vi "NEW数据采集传输系统.vi"() -> ()   [LabVIEW 2016, in "数据传输系统.lvlib"]
uses:
  <vilib>/Utility/miscctls.llb/LVPointTypeDef.ctl
  <vilib>/Utility/error.llb/whitespace.ctl
  <vilib>/Utility/config.llb/Read Key (String).vi
  <vilib>/Utility/config.llb/NI_LVConfig.lvlib
  <vilib>/Averna/Notify Icon/NotifyIcon.llb/NotifyIcon.lvclass
  <vilib>/ptbypt/NI_PtbyPt.lvlib
  <vilib>/Averna/Notify Icon/NotifyIcon.llb/BalloonIcon.ctl
  update/update.lvlib
panel:
  out "数据库打开失败次数":dbl
  out "与工控通信指示灯":bool
  in  "判断数据反馈":enum16{"非严格判断", "严格判断", "不判断"}(ring)
  in  "暂停上传":bool
  in  "参数数值":T1={"CODMn"=TRUE, "CODCr"=TRUE, "DO"=TRUE, "铜"=TRUE, "PH"=TRUE, "氨氮"=TRUE, "比电导率"=TRUE, "水温"=TRUE, "COD"=TRUE, "浊度"=TRUE, "总氮"=TRUE, "总磷"=TRUE, "叶绿素a"=TRUE, "藻密度"=TRUE, "水位"=TRUE, "流速"=TRUE, "瞬时流量"=TRUE, "累积流量"=TRUE, "亚硝氮"=TRUE, "硫化物"=TRUE, "ORP"=TRUE, "铅"=TRUE, "镉"=TRUE, "锌"=TRUE, "镍"=TRUE, "锰"=TRUE, "汞"=TRUE, "气温"=TRUE, "气压"=TRUE, "风速"=TRUE, "风向"=TRUE}
  in  "配置表":bool caption="确定"
  out "配置表格":string[][](table)
  in  "updateconfiguration":T2={"主机"="27.154.58.30", "用户"="update", "密码"="std23506", "远程路径"="数据传输系统\\平台数据传输系统.exe", "下载文件名"="平台数据传输系统.exe", "软件版本"=""}
  out "标题显示":string
  in  "更新":bool
  out "错误输出":errorcluster
  in  "系统编码选择框":string(combo)="地表水质量监测"
  in  "数据发送通道":enum16{"TCP", "VISA"}(ring)
  in  "baud rate":u32=9600 caption="波特率"
  in  "VISA resource name":refnum<visa-resource-name> caption="VISA资源名称"
  in  "实时数据发送时间间隔/min":i32=1
  in  "数据组合发送":bool
  in  "2011发送":bool
  in  "数据发送协议":enum16{"2005-212协议", "2017-212协议"}(ring)=enum."2017-212协议"
  in  "重发时间":T3(ring)
  in  "重发日期":T4(ring)
  in  "开机启动":bool
  in  "确定更改起始时间":bool
  in  "更改起始时间":bool
  in  "数据发送起始时间":timestamp format="%<%.3X\n%Y/%m/%d>T"
  in  "每周自动重发":bool=TRUE
  in  "确定":bool
  in  "返回":bool
  in  "PW":string
  in  "MN":string
  in  "PORT":string
  in  "IP":string
  in  "站点设备":string
  in  "站点名称":string
  out "设置超时时间/min":i32=1
  out "状态信息":T5={"1st Error to Convert "=63, "步骤 "=enum."发送数据", "元素"="实时数据", "TCP服务端掉线计数"=0, "TCP掉线时间节点"="2019/05/08 15:24:17"} {"1st Error to Convert" items=["无错误", "参数错误", "内存已满", "超出区域", "文件结束", "文件已打开", "一般文件IO错误", "未找到文件", "文件权限错误", "磁盘已满", "路径副本", "打开过多文件", "未启用", "未找到资源文件", "无法添加资源", "未找到资源", "未找到图像", "图像内存错误", "画笔不存在", "配置错误类型", "配置未找到解析段", "配置解析错误", "配置内存错误", "错误外部代码格式", "错误外部代码偏移量", "外部代码不存在", "空窗口", "销毁窗口错误", "空菜单", "打印已中止", "错误打印记录", "打印驱动程序错误", "打印时窗口错误", "打印时内存错误", "打印对话框错误", "一般打印错误", "无效设备引用句柄", "设备未找到", "设备参数错误", "设备单位错误", "无法打开设备", "设备调用已中止", "一般错误", "用户已取消", "对象ID过低", "对象ID过高", "对象不在堆中", "未知的堆", "错误DefProc ID", "DefProc不在表格中", "范围外信息", "空方法", "未知信息", "不支持管理器调用", "错误地址", "连接过程中", "连接超时", "连接过程中", "不支持网络属性", "网络错误", "正在使用的地址", "系统缺少内存", "连接已中止", "连接已拒绝", "连接未建立", "连接已建立", "连接已关闭", "初始化错误（交互应用程序管理器）", "错误事件发生", "等待无约束事件发生处理程序", "事件发生队列溢出", "错误路径", "未发出信号量", "未识别类型（交互应用程序管理器）"]}
  out "数据接收超时指示灯":bool
  out "空闲时间/s":string
  out "系统时间":string
  out "实时小时数据上传":bool
  out "系统状态改变":bool
  out "软件版本":string
  out "掉线指示":bool
  out "核查数据上传":bool
  out "配置信息":T6
  in  "参数配置":bool
  out "反控数据发送":bool
  out "读取报文显示":string
  out "发送报文显示":string
  out "心跳包":bool
  out "通信状态":bool
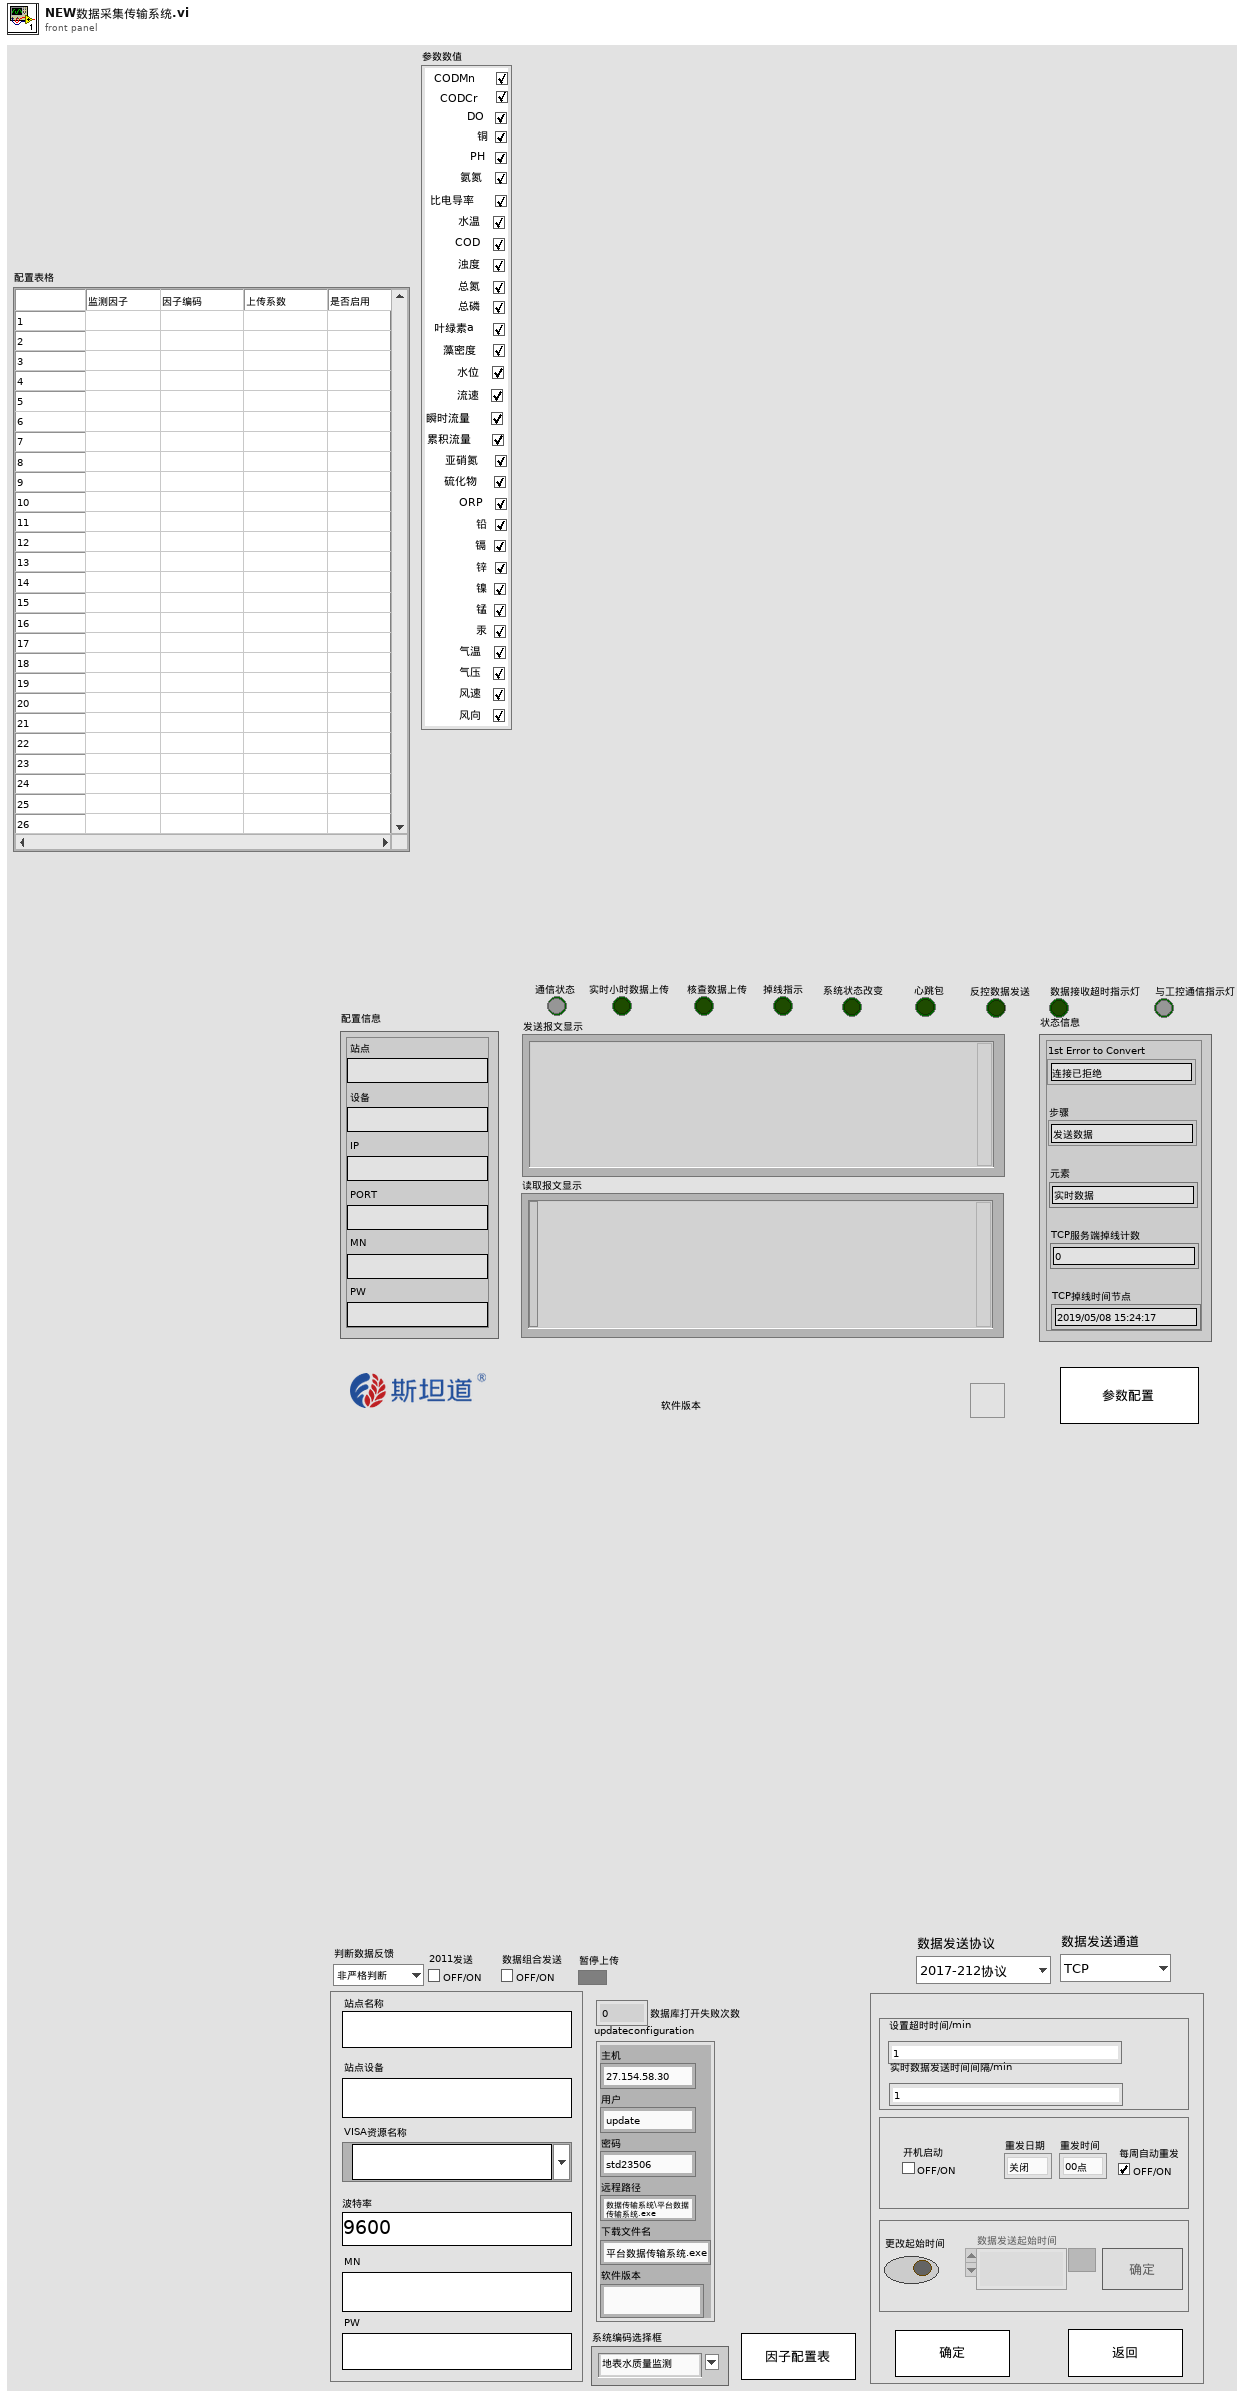
[diagram p1: front panel]
types:
  T1 = cluster{"CODMn":bool, "CODCr":bool, "DO":bool, "铜":bool, "PH":bool, "氨氮":bool, "比电导率":bool, "水温":bool, "COD":bool, "浊度":bool, "总氮":bool, "总磷":bool, "叶绿素a":bool, "藻密度":bool, "水位":bool, "流速":bool, "瞬时流量":bool, "累积流量":bool, "亚硝氮":bool, "硫化物":bool, "ORP":bool, "铅":bool, "镉":bool, "锌":bool, "镍":bool, "锰":bool, "汞":bool, "气温":bool, "气压":bool, "风速":bool, "风向":bool}
  T2 = cluster{"主机":string, "用户":string, "密码":string, "远程路径":string, "下载文件名":string, "软件版本":string}
  T3 = enum16{"00点", "01点", "02点", "03点", "04点", "05点", "06点", "07点", "08点", "09点", "10点", "11点", "12点", "13点", "14点", "15点", "16点", "17点", "18点", "19点", "20点", "21点", "22点", "23点"}
  T4 = enum16{"关闭", "星期日", "星期一", "星期二", "星期三", "星期四", "星期五", "星期六"}
  T5 = cluster{"1st Error to Convert ":i32, "步骤 ":enum16{"打开连接", "发送数据", "读取数据", "数据处理", "关闭连接"}, "元素":string, "TCP服务端掉线计数":i32, "TCP掉线时间节点":string}
  T6 = cluster{"站点":string, "设备":string, "IP":string, "PORT":string, "MN":string, "PW":string}
  T7 = cluster{"host":string, "port":u16, "user":string, "password":string, "远端地址":string}
  T8 = typedef "LVDateTimeRec.ctl" = cluster{"秒数的小数部分":dbl, "秒":i32, "分":i32, "时":i32, "日":i32, "月":i32, "年":i32, "天数（周）":i32, "天数（年）":i32, "DST":i32}
  T9 = typedef "whitespace.ctl" = u16
  T10 = typedef "LVPointTypeDef.ctl" = cluster{"Horizontal":i16, "Vertical":i16}
  T11 = cluster{"setini":string, "sysini":string, "hechaini":string, "actualwrite":string, "actualread":string, "datasent":string, "反控命令信息队列":string, "反控与仪器交互":string}
  T12 = cluster{"CODMn":string, "CODCr":string, "DO":string, "铜":string, "PH":string, "氨氮":string, "比电导率":string, "水温":string, "COD":string, "浊度":string, "总氮":string, "总磷":string, "叶绿素a":string, "藻密度":string, "水位":string, "流速":string, "瞬时流量":string, "累积流量":string, "亚硝酸盐":string, "硫化物":string, "ORP":string, "铅":string, "镉":string, "锌":string, "镍":string, "锰":string, "汞":string, "气温":string, "气压":string, "风速":string, "风向":string}
  T13 = typedef "NI_LVConfig.lvlib/Config Data RefNum.ctl" = refnum<k1>
  T14 = typedef "imagedata.ctl" = cluster{"image type":i32, "image depth":i32, "image":u8[], "mask":u8[], "colors":u32[], "Rectangle":cluster{"left":i16, "top":i16, "right":i16, "bottom":i16}}
  T15 = cluster{"[0]":string, "[1]":string, "[2]":string, "[3]":string, "[4]":string, "[5]":string, "[6]":string, "[7]":string, "[8]":string, "[9]":string, "[10]":string, "[11]":string, "[12]":string, "[13]":string, "[14]":string, "[15]":string, "[16]":string, "[17]":string, "[18]":string, "[19]":string, "[20]":string, "[21]":string, "[22]":string, "[23]":string, "[24]":string, "[25]":string, "[26]":string, "[27]":string, "[28]":string, "[29]":string, "[30]":string}
  T16 = enum8{"Enabled", "Disabled", "Disabled and Grayed Out"}
  T17 = cluster{"配置表格[0]":string, "配置表格[1]":string, "配置表格[2]":string, "配置表格[3]":string, "配置表格[4]":string, "配置表格[5]":string, "配置表格[6]":string, "配置表格[7]":string, "配置表格[8]":string, "配置表格[9]":string, "配置表格[10]":string, "配置表格[11]":string, "配置表格[12]":string, "配置表格[13]":string, "配置表格[14]":string, "配置表格[15]":string, "配置表格[16]":string, "配置表格[17]":string, "配置表格[18]":string, "配置表格[19]":string, "配置表格[20]":string, "配置表格[21]":string, "配置表格[22]":string, "配置表格[23]":string, "配置表格[24]":string, "配置表格[25]":string, "配置表格[26]":string, "配置表格[27]":string, "配置表格[28]":string, "配置表格[29]":string, "配置表格[30]":string}
  T18 = cluster{"[0]":dbl, "[1]":dbl, "[2]":dbl, "[3]":dbl, "[4]":dbl, "[5]":dbl, "[6]":dbl, "[7]":dbl, "[8]":dbl, "[9]":dbl, "[10]":dbl, "[11]":dbl, "[12]":dbl, "[13]":dbl, "[14]":dbl, "[15]":dbl, "[16]":dbl, "[17]":dbl, "[18]":dbl, "[19]":dbl, "[20]":dbl, "[21]":dbl, "[22]":dbl, "[23]":dbl, "[24]":dbl, "[25]":dbl, "[26]":dbl, "[27]":dbl, "[28]":dbl, "[29]":dbl, "[30]":dbl}
  T19 = cluster{"[0]":string, "[1]":string, "[2]":string, "[3]":string, "[4]":string, "[5]":string, "[6]":string, "[7]":string, "[8]":string, "[9]":string, "[10]":string, "[11]":string, "[12]":string}
  T20 = cluster{"[0]":string, "[1]":string, "[2]":string, "[3]":string, "[4]":string, "[5]":string, "[6]":string, "[7]":string}
  T21 = cluster{"[0]":string, "[1]":string, "[2]":string, "[3]":string, "[4]":string, "[5]":string, "[6]":string, "[7]":string, "[8]":string, "[9]":string, "[10]":string, "[11]":string, "[12]":string, "[13]":string, "[14]":string}
  T22 = cluster{"[0]":string, "[1]":string, "[2]":string, "[3]":string, "[4]":string}
  T23 = enum32{"Invalid", "Standard", "Closed", "Hidden", "Minimized", "Maximized"}
  T24 = typedef "NotifyIcon.lvlib/NotifyIcon.lvclass/BalloonIcon.ctl" = enum32{"None", "Information", "Warning", "Error"}
  T25 = enum32{"invalid app kind", "Development System", "Run Time System", "Student Edition", "Embedded LabVIEW", "Evaluation", "Custom"}
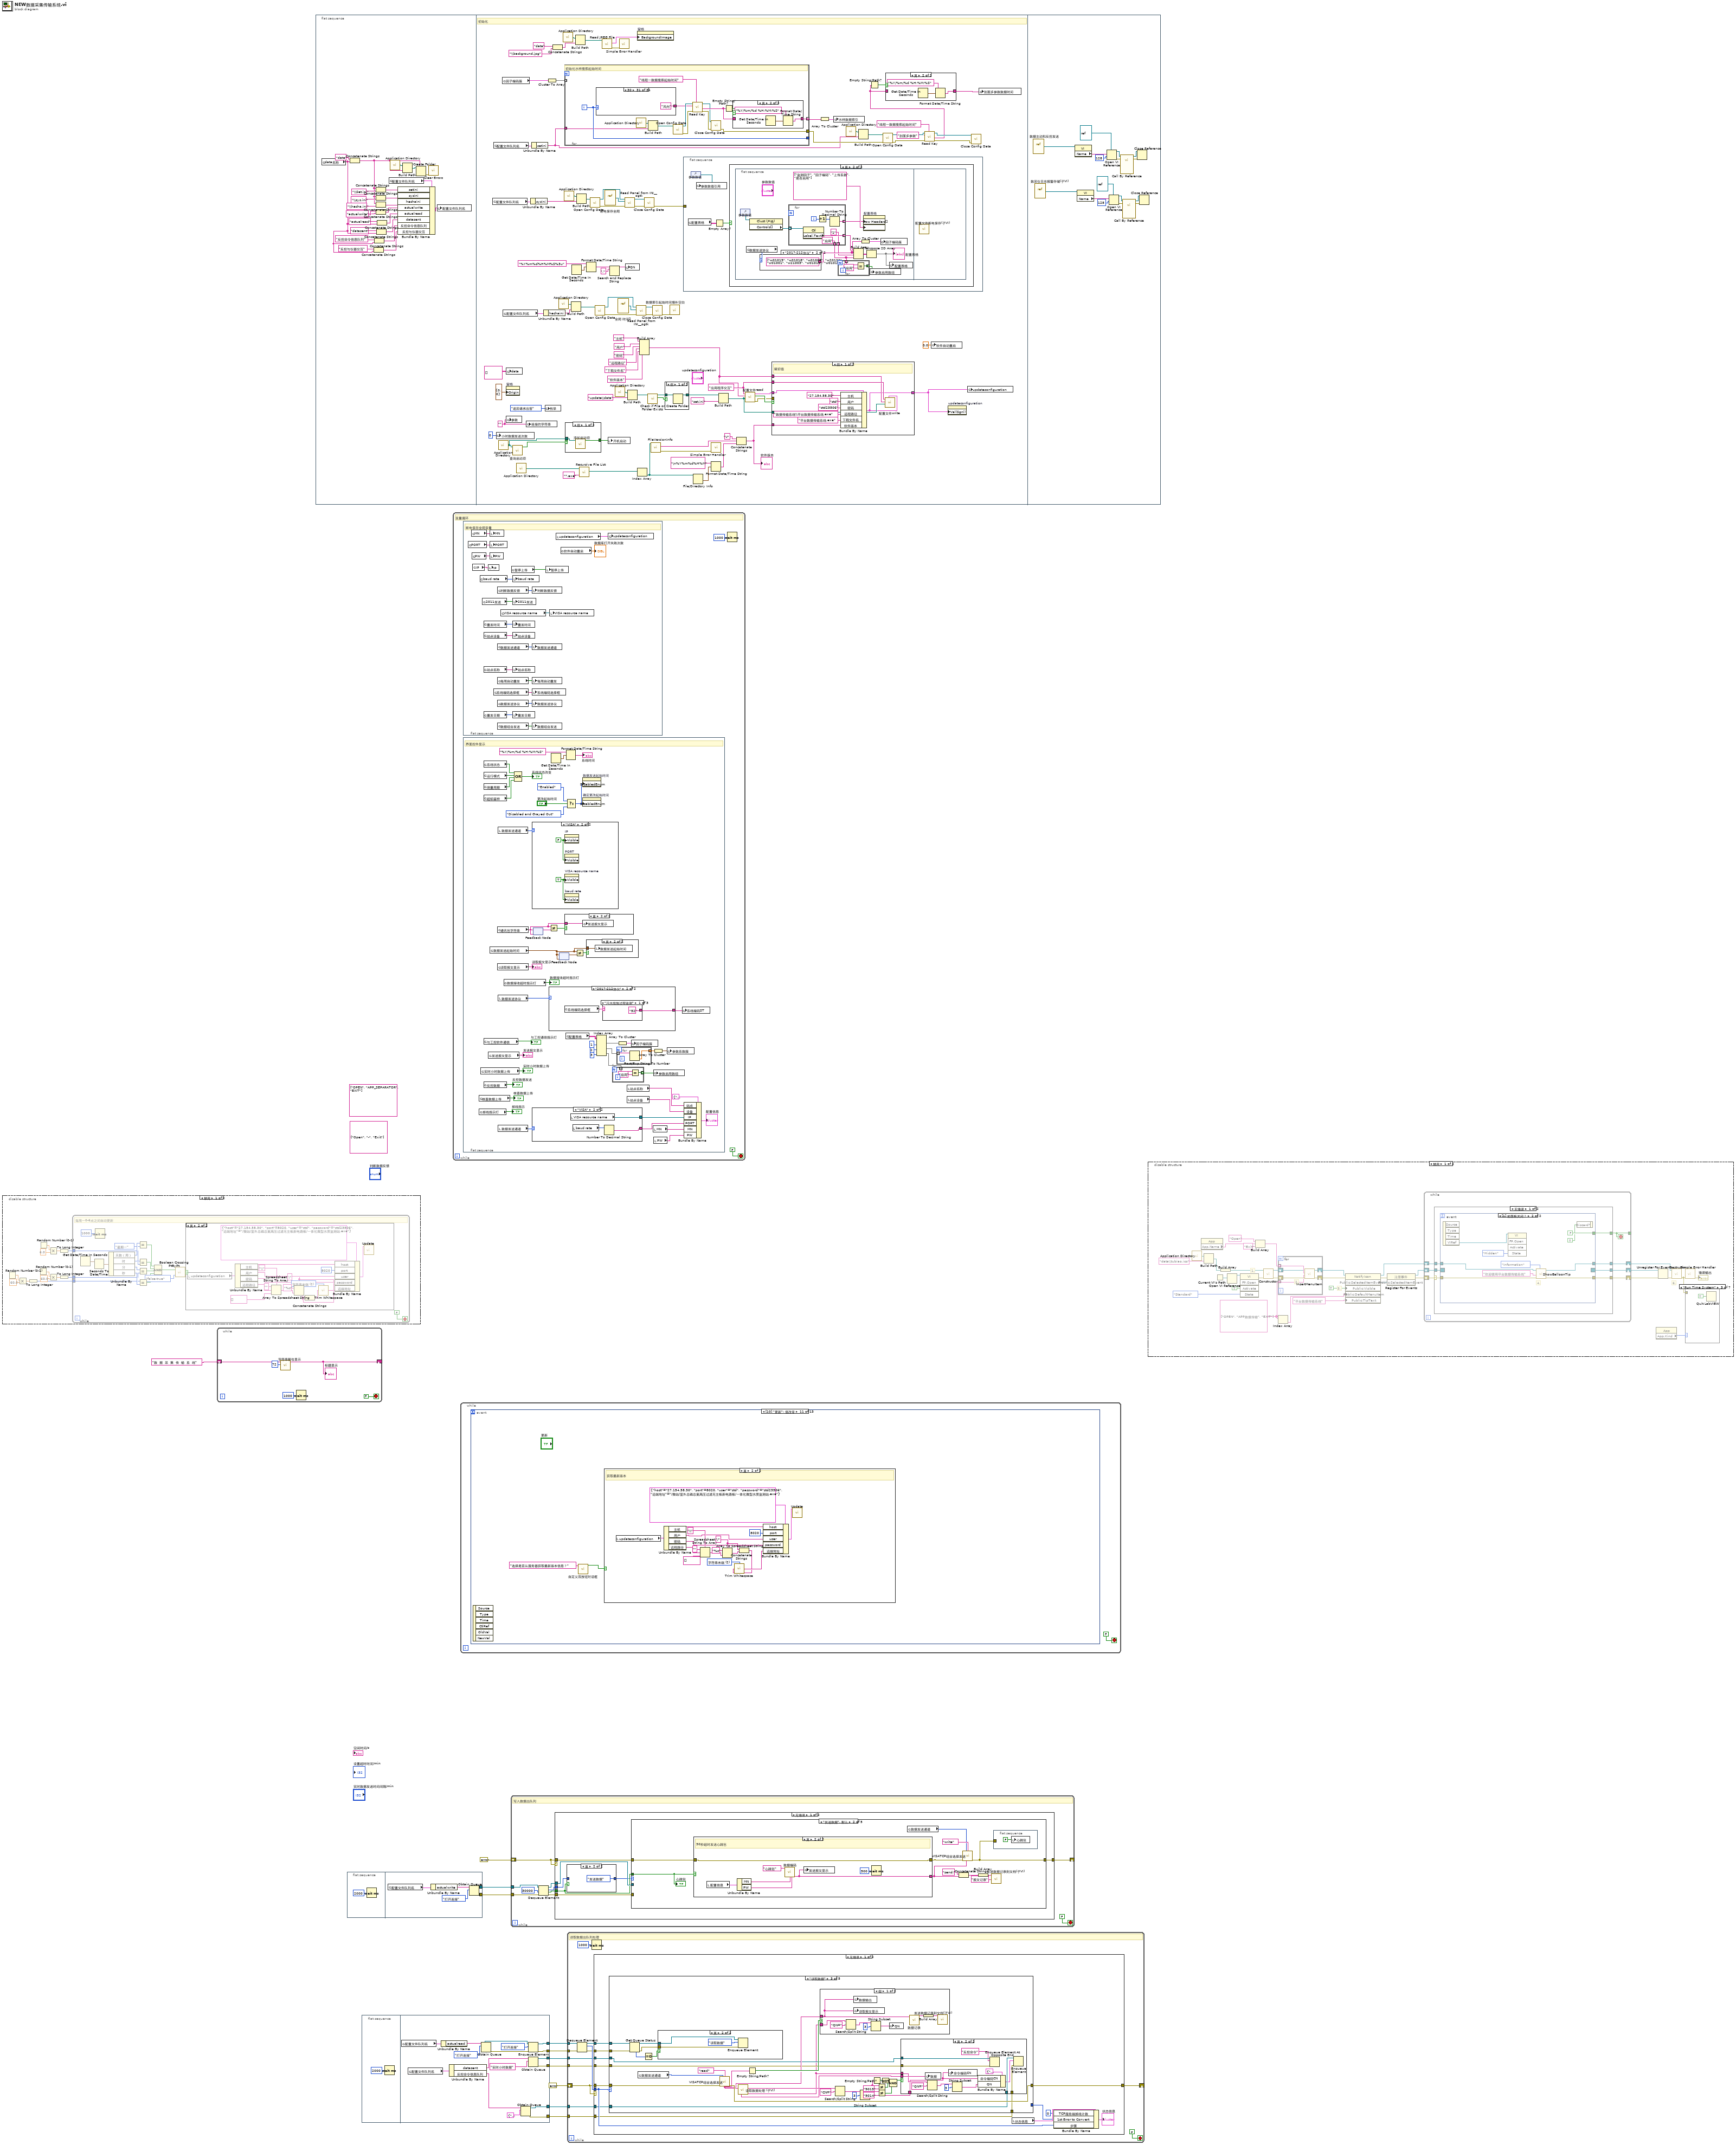
[diagram p0: block diagram]
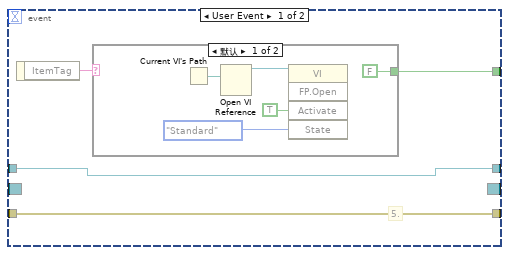
[diagram p4: hidden frame]
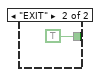
[diagram p5: hidden frame]
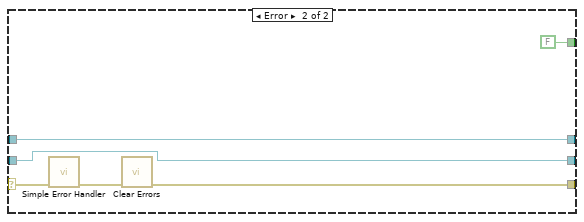
[diagram p6: hidden frame]
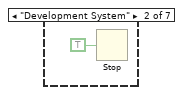
[diagram p8: hidden frame]
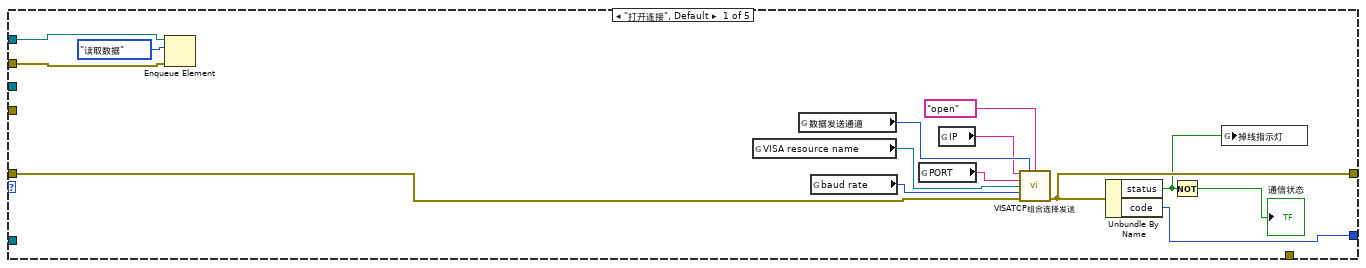
[diagram p14: hidden frame]
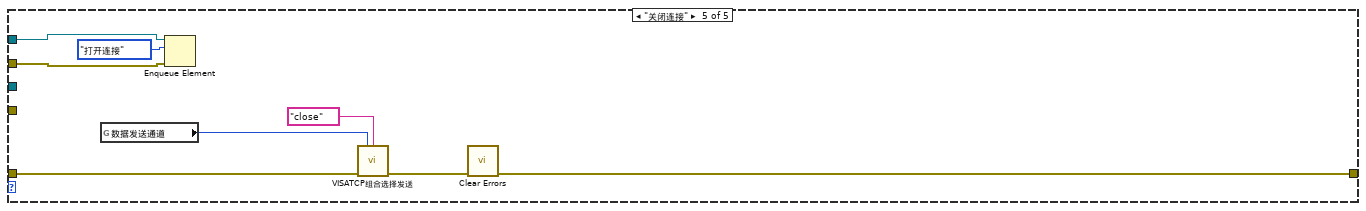
[diagram p20: hidden frame]
diagram:
  (unwired) string[] ["OPEN", "APP_SEPARATOR", "EXIT"]
  (unwired) string[] ["Open", "-", "Exit"]
  n1 = disable-structure shown="禁用" {
    frame Disabled {
      n2 = Random Number (0-1)() -> (number: 0 to 1=w19:dbl)
      n3 = Multiply(x=w19, y=60.0) -> (x*y=w13:dbl)
      n4 = To Long Integer(number=w13) -> (32bit integer=w12:i32)
      n5 = Random Number (0-1)() -> (number: 0 to 1=w20:dbl)
      n6 = Random Number (0-1)() -> (number: 0 to 1=w23:dbl)
      n7 = Multiply(x=w23, y=6.0) -> (x*y=w17:dbl)
      n8 = Multiply(x=w20, y=60.0) -> (x*y=w15:dbl)
      n9 = To Long Integer(number=w17) -> (32bit integer=w16:i32)
      n10 = To Long Integer(number=w15) -> (32bit integer=w14:i32)
      n11 = while {
        tunnel: w16 -> [w31]
        tunnel: w14 -> [w26]
        tunnel: w12 -> [w25]
        stop <- FALSE stop-if-true
        # "每周一0-6点之间自动更新"
        n12 = Get Date/Time In Seconds() -> (seconds since 1Jan1904=w40:timestamp)
        n13 = Seconds To Date/Time(time stamp (now)=w40) -> (date time rec=w36:T8)  [unwired: 1 in]
        n14 = Wait (ms)(milliseconds to wait=u32 1000 ("等待时间（毫秒）")) -> ()  [unwired: 1 out]
        n15 = Unbundle By Name(w36) -> ("天数（周）"=w39:i32, "时"=w33:i32, "分"=w30:i32, "秒"=w28:i32)
        n16 = Equal?(x=w39, y=T4."星期一" ("重发日期")) -> (x = y?=w38:bool)
        n17 = Equal?(x=w33, y=w31) -> (x = y?=w37:bool)
        n18 = Equal?(x=w30, y=w26) -> (x = y?=w29:bool)
        n19 = Equal?(x=w25, y=w28) -> (x = y?=w27:bool)
        n20 = Compound Arithmetic op=AND ("复合运算")(w38, w37, w29, w27) -> (w35:bool)
        n21 = call <vilib>:"Boolean Crossing PtByPt.vi"("direction"=enum16{"either", "false-true", "true-false"}."false-true", "input"=w35) -> ("crossing"=w24:bool)  [unwired: 1 in]
        n22 = case shown="真" w24 {
          frame False {
          }
          frame True {
            w48 = T9 2 items=["两端", "字符串首端", "字符串末端"] ("location (both)")
            w45 = "/" ("分隔符(Tab)")
            n23 = local read "updateconfiguration"() -> (w58:T2)
            n24 = Unbundle By Name(w58) -> ("主机"=w57:string, "用户"=w56:string, "密码"=w55:string, "远程路径"=w53:string)
            n25 = Spreadsheet String To Array(delimiter (Tab)="\\" ("分隔符(Tab)"), format string="" ("格式字符串"), spreadsheet string=w53, array type (2D Dbl)=string[] []) -> (array=w50:string[])
            n26 = Array To Spreadsheet String(delimiter (Tab)=w45, array=w50, 3:"%s" ("格式字符串")) -> (spreadsheet string=w44:string)
            n27 = Concatenate Strings(w45, w44) -> (w43:string)
            n28 = call <vilib>:"Trim Whitespace.vi"("string"=w43, "location (both)"=w48) -> ("trimmed string"=w47:string)
            n29 = Bundle By Name(cluster=T7 {"host"="27.154.58.30", "port"=8020, "user"="std", "password"="std23506", "远端地址"="/微站/室外总磷总氮高压过滤无主板新电路板/一体化微型水质监测站.exe"} ("服务器信息"), "host"=w57, "port"=u16 8020, "user"=w56, "password"=w55, "远端地址"=w47) -> (w59:T7)
            n30 = call "Update.vi"("服务器信息"=w59) -> ()  [unwired: 11 in]
          }
        }
      }
    }
    frame Enabled {
    }
  }
  n31 = while {
    shift-right: [w62] -> _
    shift-left: "数  据  采  集  传  输  系  统" ("标题显示") -> [w63]
    stop <- FALSE stop-if-true
    n32 = call "字符串移位显示.vi"("字符框大小"=72, "字符串输入"=w63) -> ("移位后字符串"=w62:string)  [unwired: 8 in, 1 out]
    "标题显示" <- w62
    n33 = Wait (ms)(milliseconds to wait=u32 1000 ("等待时间（毫秒）")) -> ()  [unwired: 1 out]
  }
  n34 = flat-sequence {
    frame #0 {
      n35 = global read "断电保存全局.vi" "data名称"() -> (w68:string)
      n36 = Concatenate Strings("data" ("对话框窗口（创建文件夹）"), w68) -> (w82:string)
      n37 = Concatenate Strings("反控与仪器交互" ("名称（未命名）"), w68) -> (w67:string)
      n38 = Concatenate Strings("反控命令信息队列" ("名称（未命名）"), w68) -> (w66:string)
      n39 = Concatenate Strings(w82, "\\Set.ini" ("名称或相对路径")) -> (w84:string)
      n40 = Concatenate Strings(w82, "\\sys.ini" ("名称或相对路径")) -> (w81:string)
      n41 = Concatenate Strings(w82, "\\hecha.ini" ("名称或相对路径")) -> (w80:string)
      n42 = Concatenate Strings("actualwrite" ("名称（未命名）"), w68) -> (w77:string)
      n43 = Concatenate Strings("datasent" ("名称（未命名）"), w68) -> (w73:string)
      n44 = Concatenate Strings("actualread" ("名称（未命名）"), w68) -> (w75:string)
      n45 = global read "断电保存全局.vi" "配置文件队列名"() -> (w72:T11)
      n46 = call <vilib>:"Application Directory.vi"() -> ("Application Directory"=w88:path)
      n47 = Bundle By Name(cluster=w72, "setini"=w84, "sysini"=w81, "hechaini"=w80, "actualwrite"=w77, "actualread"=w75, "datasent"=w73, "反控命令信息队列"=w66, "反控与仪器交互"=w67) -> (w71:T11)
      n48 = Build Path(base path=w88, name or relative path=w82) -> (appended path=w87:path)
      n49 = Create Folder(prompt (Create Folder)=w82, path (use dialog)=w87) -> (error out=w86:errorcluster)  [unwired: 1 in, 2 out]
      n50 = call <vilib>:"Clear Errors.vi"("error in (no error)"=w86) -> ()  [unwired: 5 in, 2 out]
      n51 = global write "断电保存全局.vi" "配置文件队列名"(w71) -> ()
    }
    frame #1 {
      w133 = "应用程序交互" ("section")
      w177 = "" ("参数")
      # "初始化"
      n52 = global read "断电保存全局.vi" "配置文件队列名"() -> (w94:T11)
      n53 = global read "断电保存全局.vi" "配置文件队列名"() -> (w96:T11)
      n54 = global write "全局 小时数据发送次数.vi" "小时数据发送次数"(0 ("数值")) -> ()
      n55 = call <vilib>:"Application Directory.vi"() -> ("Application Directory"=w104:path)
      n56 = global read "断电保存全局.vi" "因子编码簇"() -> (w101:T12)
      n57 = global read "断电保存全局.vi" "配置文件队列名"() -> (w92:T11)
      n58 = global write "全局 实时数据参数.vi" "data"(string[][] [] ("data")) -> ()
      n59 = property on="窗格" class="Pane"("Origin"=T10 {"Horizontal"=0, "Vertical"=0} ("原点")) -> ()  [unwired: 2 in, 2 out]
      n60 = global write "全局 实时数据参数.vi" "参数"(w177) -> ()
      n61 = call "查询启动项.vi"("启动文件路径"=w104) -> ("包含启动项"=w105:bool)  [unwired: 9 in, 1 out]
      n62 = call <vilib>:"Application Directory.vi"() -> ("Application Directory"=w158:path)
      n63 = global write "全局 实时数据参数.vi" "连接的字符串"(w177) -> ()
      n64 = Unbundle By Name(w94) -> ("sysini"=w93:string)
      n65 = Unbundle By Name(w96) -> ("setini"=w95:string)
      n66 = Unbundle By Name(w92) -> ("hechaini"=w91:string)
      n67 = global write "全局1.vi" "枚举"(enum16{"返回请求应答", "上传数据", "返回执行结果"}."返回请求应答" ("枚举")) -> ()
      n68 = Cluster To Array(cluster=w101) -> (array=w139:string[])
      n69 = Concatenate Strings("data" ("名称或相对路径"), "\\background.jpg" ("名称或相对路径")) -> (w98:string)
      n70 = call <vilib>:"Application Directory.vi"() -> ("Application Directory"=w146:path)
      n71 = call <vilib>:"Application Directory.vi"() -> ("Application Directory"=w169:path)
      n72 = call <vilib>:"Application Directory.vi"() -> ("Application Directory"=w152:path)
      n73 = for {
        tunnel: w139 -> [_] mode=indexing
        tunnel: [w242] -> _
        tunnel: [w239] -> w138 mode=indexing
        tunnel: [w238] -> w115
        tunnel: w95 -> [w237]
        i -> [w242]
        # "初始化水样搜索起始时间"
        n74 = case shown="30" w242 {
          tunnel: ["CODMn" "CODCr" "DO" "铜" "PH" "氨氮" "比电导率" "水温" "COD" "浊度" "总氮" "总磷" "叶绿素a" "藻密度" "水位" "流速" "瞬时流量" "累积流量" "亚硝氮" "硫化物" "ORP" "铅" "镉" "锌" "镍" "锰" "汞" "气温" "气压" "风速" "风向"] -> w245
          frame 0, Default {
          }
          frame 1 {
          }
          frame 2 {
          }
          frame 3 {
          }
          frame 4 {
          }
          frame 5 {
          }
          frame 6 {
          }
          frame 7 {
          }
          frame 8 {
          }
          frame 9 {
          }
          frame 10 {
          }
          frame 11 {
          }
          frame 12 {
          }
          frame 13 {
          }
          frame 14 {
          }
          frame 15 {
          }
          frame 16 {
          }
          frame 17 {
          }
          frame 18 {
          }
          frame 19 {
          }
          frame 20 {
          }
          frame 21 {
          }
          frame 22 {
          }
          frame 23 {
          }
          frame 24 {
          }
          frame 25 {
          }
          frame 26 {
          }
          frame 27 {
          }
          frame 28 {
          }
          frame 29 {
          }
          frame 30 {
          }
        }
        n75 = call <vilib>:"Application Directory.vi"() -> ("Application Directory"=w250:path)
        n76 = Build Path(base path=w250, name or relative path=w237) -> (appended path=w249:path)
        n77 = call <vilib>:"Open Config Data.vi"("configuration file path"=w249) -> ("error out"=w247:errorcluster, "refnum"=w248:T13)  [unwired: 8 in, 1 out]
        n78 = call-poly <vilib>:"Read Key.vi"("section"="线程一数据搜索起始时间", "error in (no error)"=w247, "key"=w245, "refnum"=w248) -> ("error out"=w240:errorcluster, "value"=w243:string, "refnum out"=w241:T13)  [unwired: 4 in, 1 out]
        n79 = call <vilib>:"Close Config Data.vi"("error in (no error)"=w240, "refnum"=w241) -> ("error out"=w238:errorcluster)  [unwired: 8 in, 1 out]
        n80 = Empty String/Path?(string/path=w243) -> (empty?=w244:bool)
        n81 = case shown="真" w244 {
          tunnel: [w251 w252] -> w239
          tunnel: w243 -> [w251 _]
          frame False {
          }
          frame True {
            n82 = Get Date/Time In Seconds() -> (seconds since 1Jan1904=w254:timestamp)
            n83 = Format Date/Time String(time format string (%c)="%Y/%m/%d %H:%M:%S" ("时间格式字符串(%c)"), seconds (now)=w254) -> (date/time string=w252:string)  [unwired: 1 in]
          }
        }
      }
      n84 = case shown="假" w105 {
        selector: w105 -> [_ w210]
        tunnel: w104 -> [w209 _]
        tunnel: [w208 w210] -> w103
        frame False {
          n85 = call "添加启动项.vi"("启动文件路径"=w209) -> ("添加成功标记"=w208:bool)  [unwired: 9 in, 1 out]
        }
        frame True {
        }
      }
      n86 = Build Path(base path=w146, name or relative path=w91) -> (appended path=w147:path)
      n87 = Get Date/Time In Seconds() -> (seconds since 1Jan1904=w173:timestamp)
      n88 = Build Path(base path=w169, name or relative path=w98) -> (appended path=w168:path)
      n89 = Build Path(base path=w152, name or relative path=w93) -> (appended path=w151:path)
      n90 = call <vilib>:"Recursive File List.vi"("pattern"="*.exe", "Folder Path"=w158) -> ("All Files in Dir"=w164:path[])  [unwired: 5 in, 4 out]
      n91 = Format Date/Time String(time format string (%c)="%Y%m%d%H%M%S%3u" ("时间格式字符串(%c)"), seconds (now)=w173) -> (date/time string=w172:string)  [unwired: 1 in]
      n92 = call <vilib>:"Open Config Data.vi"("configuration file path"=w151) -> ("error out"=w156:errorcluster, "refnum"=w155:T13)  [unwired: 8 in, 1 out]
      n93 = call <vilib>:"Open Config Data.vi"("configuration file path"=w147) -> ("error out"=w142:errorcluster, "refnum"=w143:T13)  [unwired: 8 in, 1 out]
      n94 = call <vilib>:"Read JPEG File.vi"("path to JPEG file"=w168) -> ("error out"=w166:errorcluster, "image data"=w167:T14)  [unwired: 8 in, 1 out]
      n95 = vi-ref "断电保存全局.vi"() -> (w154:refnum<vi>)
      n96 = local write "开机启动"(w103) -> ()
      n97 = Search and Replace String(input string=w172, search string="." ("搜索字符串")) -> (result string=w170:string)  [unwired: 6 in, 3 out]
      n98 = call <vilib>:"Application Directory.vi"() -> ("Application Directory"=w120:path)
      n99 = vi-ref "全局 时间2.vi"() -> (w144:refnum<vi>)
      n100 = call <vilib>:"Simple Error Handler.vi"("error in (no error)"=w166) -> ()  [unwired: 4 in, 5 out]
      n101 = call <userlib>:"Read Panel from INI__ogtk.vi"("error in (no error)"=w156, "VI ref"=w154, "refnum"=w155) -> ("error out"=w150:errorcluster, "refnum out"=w153:T13)  [unwired: 7 in]
      n102 = global write "全局1.vi" "QN"(w170) -> ()
      n103 = Build Path(base path=w120, name or relative path="update\\data" ("名称或相对路径")) -> (appended path=w121:path)
      n104 = call <userlib>:"Read Panel from INI__ogtk.vi"("error in (no error)"=w142, "VI ref"=w144, "refnum"=w143) -> ("error out"=w141:errorcluster, "refnum out"=w145:T13)  [unwired: 7 in]
      n105 = property on="窗格" class="Pane"("BackgroundImage"=w167) -> ()  [unwired: 2 in, 2 out]
      n106 = Index Array(array=w164) -> (element=w163:path)  [unwired: 1 in]
      n107 = Build Array("主机" ("section"), "用户" ("section"), "密码" ("key"), "远程路径" ("key"), "下载文件名" ("key"), "软件版本" ("key")) -> (w124:string[])
      n108 = call <vilib>:"Close Config Data.vi"("error in (no error)"=w150, "refnum"=w153) -> ("error out"=w102:errorcluster)  [unwired: 8 in, 1 out]
      n109 = call <vilib>:"Check if File or Folder Exists.vi"("path"=w121) -> ("file or folder exists?"=w122:bool, "dup path"=w123:path)  [unwired: 8 in, 1 out]
      n110 = call <vilib>:"FileVersionInfo.vi"("Application Path in"=w163) -> ("error out"=w157:errorcluster, "File Version Info"=w148:string)  [unwired: 7 in, 2 out]
      n111 = call <vilib>:"Close Config Data.vi"("error in (no error)"=w141, "refnum"=w145) -> ("error out"=w140:errorcluster)  [unwired: 8 in, 1 out]
      n112 = case shown="假" w122 {
        tunnel: w123 -> [w216 w217]
        tunnel: [w215 w217] -> w118
        frame False {
          n113 = Create Folder(path (use dialog)=w216) -> (created path=w215:path)  [unwired: 2 in, 2 out]
        }
        frame True {
        }
      }
      n114 = call "数据索引起始时间填补空白.vi"("error in (no error)"=w140) -> ()  [unwired: 10 in, 1 out]
      n115 = flat-sequence {
        tunnel: w102 -> [_]
        frame #0 {
          n116 = global read "断电保存全局.vi" "配置表格"() -> (w182:string[][])
          n117 = control-ref of="参数数值"() -> (w180:refnum<vi>)
          n118 = global write "断电保存全局.vi" "参数数值引用"(w180) -> ()
          n119 = Empty Array?(array=w182) -> (empty?=w181:bool)
          n120 = case shown="真" w181 {
            frame False {
            }
            frame True {
              n121 = flat-sequence {
                frame #0 {
                  n122 = control-ref of="参数数值"() -> (w185:refnum<vi>)
                  n123 = global read "断电保存全局.vi" "数据发送协议"() -> (w189:enum16{"2005-212协议", "2017-212协议"})
                  n124 = property on="属性节点" class="Clust (严格)"(reference=w185) -> ("Controls[]"=w191:refnum<vi>[])  [unwired: 1 in, 2 out]
                  n125 = case shown="\"2017-212协议\"" w189 {
                    tunnel: [string[] ["w01019", "011", "w01009", "w20122", "001", "060", "w01014", "w01010", "w01018", "w01003", "065", "101", "w01016", "w19011", "e01201", "e01202", "B01", "e01204", "w21006", "w21019", "w01100", "w20120", "w20115", "w20123", "w20121", "w20124", "w20111"] string[] ["w01019", "w01018", "w01009", "w20122", "w01001", "w21003", "w01014", "w01010", "w01018", "w01003", "w21001", "w21011", "w01016", "w19011", "e01201", "e01202", "e01203", "e01204", "w21006", "w21019", "w01100", "w20120", "w20115", "w20123", "w20121", "w20124", "w20111"]] -> w187
                    frame "2005-212协议", Default {
                    }
                    frame "2017-212协议" {
                    }
                  }
                  n126 = for {
                    tunnel: w191 -> [w207] mode=indexing
                    tunnel: [w206] -> w193 mode=indexing
                    tunnel: [w204] -> w192 mode=indexing
                    tunnel: ["1"] -> w186 mode=indexing
                    tunnel: ["启用"] -> w184 mode=indexing
                    i -> [w205]
                    n127 = property class="Ctl"(reference=w207) -> ("Label.Text"=w206:string)  [unwired: 1 in, 2 out]
                    n128 = Increment(x=w205) -> (x+1=w203:i32)
                    n129 = Number To Decimal String(number=w203) -> (decimal integer string=w204:string)  [unwired: 1 in]
                  }
                  n130 = for {
                    tunnel: w184 -> [w198] mode=indexing
                    tunnel: [w196] -> w183 mode=indexing
                    n131 = Equal?(x=w198, y="启用") -> (x = y?=w196:bool)
                  }
                  n132 = Build Array(w193, w187, w186, w184) -> (w195:string[][])
                  n133 = Array To Cluster(array=w187) -> (cluster=w188:T15)
                  n134 = property on="配置表格" class="Tbl (严格)"("Row Headers[]"=w192, "Column Headers[]"=string[] ["监测因子", "因子编码", "上传系数", "是否启用"]) -> ()  [unwired: 2 in, 2 out]
                  n135 = Transpose 2D Array(2D array=w195) -> (transposed array=w190:string[][])
                  "配置表格" <- w190
                  n136 = global write "断电保存全局.vi" "参数启用数组"(w183) -> ()
                  n137 = global write "断电保存全局.vi" "因子编码簇"(w188) -> ()
                  n138 = global write "断电保存全局.vi" "配置表格"(w190) -> ()
                }
                frame #1 {
                  n139 = call "配置文件断电保存(子VI).vi"() -> ()  [unwired: 12 in]
                }
              }
            }
          }
        }
      }
      n140 = File/Directory Info(path=w163) -> (last mod=w162:timestamp)  [unwired: 1 in, 6 out]
      n141 = call <vilib>:"Simple Error Handler.vi"("error in (no error)"=w157) -> ()  [unwired: 4 in, 5 out]
      n142 = Format Date/Time String(time format string (%c)="\n%Y%m%d%H%M" ("时间格式字符串(%c)"), seconds (now)=w162) -> (date/time string=w159:string)  [unwired: 1 in]
      n143 = Build Path(base path=w118, name or relative path="set.ini" ("名称或相对路径")) -> (appended path=w132:path)
      n144 = Concatenate Strings("V" ("字符串"), w148, w159) -> (w134:string)
      "软件版本" <- w134
      n145 = call "配置文件read.vi"("configuration file path"=w132, "键数组"=w124, "段"=w133) -> ("error out"=w131:errorcluster, "section exists?"=w136:bool, "updateconfiguration"=w135:T2)  [unwired: 6 in]
      n146 = case shown="假" w136 {
        tunnel: w135 -> [w224 w231]
        tunnel: [w223 w230] -> w90
        tunnel: w134 -> [w218 w236]
        tunnel: w133 -> [w227 w235]
        tunnel: w124 -> [w226 w234]
        tunnel: w132 -> [w225 w233]
        tunnel: w131 -> [_ w232]
        frame False {
          # "赋初值"
          n147 = Bundle By Name(cluster=w224, "主机"="27.154.58.30" ("key"), "用户"="std", "密码"="std23506", "远程路径"="数据传输系统\\平台数据传输系统.exe", "下载文件名"="平台数据传输系统.exe", "软件版本"=w218) -> (w223:T2)
          n148 = call "配置文件write.vi"("updateconfiguration"=w223, "configuration file path"=w225, "键数组"=w226, "段"=w227) -> ()  [unwired: 7 in, 1 out]
        }
        frame True {
          # "本地"
          n149 = Bundle By Name(cluster=w231, "用户"="std", "软件版本"=w236) -> (w230:T2)
          n150 = call "配置文件write.vi"("updateconfiguration"=w230, "error in (no error)"=w232, "configuration file path"=w233, "键数组"=w234, "段"=w235) -> ()  [unwired: 6 in, 1 out]
        }
      }
      n151 = Array To Cluster(array=w138) -> (cluster=w137:T15)
      n152 = global write "全局 水样时间.vi" "水样数据索引"(w137) -> ()
      n153 = call <vilib>:"Application Directory.vi"() -> ("Application Directory"=w117:path)
      n154 = Build Path(base path=w117, name or relative path=w95) -> (appended path=w116:path)
      n155 = call <vilib>:"Open Config Data.vi"("error in (no error)"=w115, "configuration file path"=w116) -> ("error out"=w112:errorcluster, "refnum"=w113:T13)  [unwired: 7 in, 1 out]
      n156 = call-poly <vilib>:"Read Key.vi"("section"="线程一数据搜索起始时间", "error in (no error)"=w112, "key"="剖面多参数", "refnum"=w113) -> ("error out"=w109:errorcluster, "value"=w107:string, "refnum out"=w110:T13)  [unwired: 4 in, 1 out]
      n157 = Empty String/Path?(string/path=w107) -> (empty?=w106:bool)
      n158 = case shown="真" w106 {
        tunnel: [w211 w212] -> w108
        tunnel: w107 -> [w211 _]
        frame False {
        }
        frame True {
          n159 = Get Date/Time In Seconds() -> (seconds since 1Jan1904=w214:timestamp)
          n160 = Format Date/Time String(time format string (%c)="%Y/%m/%d %H:%M:%S" ("时间格式字符串(%c)"), seconds (now)=w214) -> (date/time string=w212:string)  [unwired: 1 in]
        }
      }
      n161 = global write "全局1.vi" "软件自动重启"(0.0 ("软件自动重启")) -> ()
      n162 = property on="updateconfiguration" class="Clust (严格)"("Val(Sgnl)"=w90) -> ()  [unwired: 2 in, 2 out]
      n163 = global write "update全局.vi" "updateconfiguration"(w90) -> ()
      n164 = call <vilib>:"Close Config Data.vi"("error in (no error)"=w109, "refnum"=w110) -> ()  [unwired: 8 in, 2 out]
      n165 = global write "全局 水样时间.vi" "剖面多参数数据时间"(w108) -> ()
    }
    frame #2 {
      n166 = vi-ref "数据主动和反控发送.vi"() -> (w293:refnum<vi>)
      n167 = vi-ref "数采仪日志报警存储(子VI).vi"() -> (w294:refnum<vi>)
      n168 = property class="VI"(reference=w293) -> ("Name"=w292:string)  [unwired: 1 in, 2 out]
      n169 = property class="VI"(reference=w294) -> ("Name"=w301:string)  [unwired: 1 in, 2 out]
      n170 = Open VI Reference(type specifier VI Refnum (for type only)=refnum<vi> refnum, vi path=w292, options=128 ("选项")) -> (vi reference=w290:refnum<vi>, error out=w288:errorcluster)  [unwired: 3 in]
      n171 = Open VI Reference(type specifier VI Refnum (for type only)=refnum<vi> refnum, vi path=w301, options=128 ("选项")) -> (vi reference=w299:refnum<vi>, error out=w297:errorcluster)  [unwired: 3 in]
      n172 = call-by-ref "?"(reference=w290, error in=w288) -> (reference out=w286:refnum<vi>, error out=w287:errorcluster)  [unwired: 12 in]
      n173 = call-by-ref "?"(reference=w299, error in=w297) -> (reference out=w295:refnum<vi>, error out=w296:errorcluster)  [unwired: 12 in]
      n174 = Close Reference(reference=w286, error in (no error)=w287) -> ()  [unwired: 1 out]
      n175 = Close Reference(reference=w295, error in (no error)=w296) -> ()  [unwired: 1 out]
    }
  }
  n176 = flat-sequence {
    tunnel: [w306] -> w11
    tunnel: [w305] -> w10
    frame #0 {
      n177 = Wait (ms)(milliseconds to wait=u32 2000 ("等待时间（毫秒）")) -> ()  [unwired: 1 out]
    }
    frame #1 {
      n178 = global read "断电保存全局.vi" "配置文件队列名"() -> (w304:T11)
      n179 = Unbundle By Name(w304) -> ("actualwrite"=w303:string)
      n180 = Obtain Queue(name (unnamed)=w303, element data type=enum16{"打开连接", "发送数据", "读取数据", "数据处理", "关闭连接"}."打开连接" ("枚举")) -> (queue out=w306:refnum<queue>, error out=w305:errorcluster)  [unwired: 3 in, 1 out]
    }
  }
  n181 = flat-sequence {
    tunnel: [w322] -> w8
    tunnel: [w321] -> w7
    tunnel: [w319] -> w5
    tunnel: [w318] -> w4
    tunnel: [w316] -> w3
    tunnel: [w315] -> w2
    frame #0 {
      n182 = Wait (ms)(milliseconds to wait=u32 2000 ("等待时间（毫秒）")) -> ()  [unwired: 1 out]
    }
    frame #1 {
      n183 = global read "断电保存全局.vi" "配置文件队列名"() -> (w313:T11)
      n184 = global read "断电保存全局.vi" "配置文件队列名"() -> (w311:T11)
      n185 = Unbundle By Name(w313) -> ("actualread"=w312:string)
      n186 = Unbundle By Name(w311) -> ("datasent"=w310:string, "反控命令信息队列"=w309:string)
      n187 = Obtain Queue(name (unnamed)=w312, element data type=enum16{"打开连接", "发送数据", "读取数据", "数据处理", "关闭连接"}."打开连接" ("枚举")) -> (queue out=w325:refnum<queue>, error out=w320:errorcluster)  [unwired: 3 in, 1 out]
      n188 = Obtain Queue(name (unnamed)=w309, element data type=cluster{"命令编码CN":string, "QN":string} {"命令编码CN"="", "QN"=""}) -> (queue out=w316:refnum<queue>, error out=w315:errorcluster)  [unwired: 3 in, 1 out]
      n189 = Enqueue Element(queue=w325, element=enum16{"打开连接", "发送数据", "读取数据", "数据处理", "关闭连接"}."打开连接" ("枚举"), error in (no error)=w320) -> (queue out=w322:refnum<queue>, error out=w321:errorcluster)  [unwired: 1 in, 1 out]
      n190 = Obtain Queue(name (unnamed)=w310, element data type="实时小时数据" ("元素")) -> (queue out=w319:refnum<queue>, error out=w318:errorcluster)  [unwired: 3 in, 1 out]
    }
  }
  n191 = while {
    stop <- FALSE stop-if-true
    # "变量循环"
    n192 = flat-sequence {
      frame #0 {
        # "断电保存全局变量"
        n193 = global read "断电保存全局.vi" "PORT"() -> (w415:string)
        n194 = global read "断电保存全局.vi" "MN"() -> (w414:string)
        n195 = global read "断电保存全局.vi" "PW"() -> (w413:string)
        n196 = global read "断电保存全局.vi" "IP"() -> (w416:string)
        n197 = global read "断电保存全局.vi" "baud rate"() -> (w411:u32)
        n198 = global read "断电保存全局.vi" "2011发送"() -> (w407:bool)
        n199 = global read "断电保存全局.vi" "重发时间"() -> (w402:T3)
        n200 = global read "断电保存全局.vi" "站点设备"() -> (w417:string)
        n201 = global read "断电保存全局.vi" "站点名称"() -> (w418:string)
        n202 = global read "断电保存全局.vi" "重发日期"() -> (w409:T4)
        n203 = local write "IP"(w416) -> ()
        n204 = local write "MN"(w414) -> ()
        n205 = local write "PORT"(w415) -> ()
        n206 = local write "PW"(w413) -> ()
        n207 = global read "断电保存全局.vi" "系统编码选择框"() -> (w403:string)
        n208 = global read "断电保存全局.vi" "判断数据反馈"() -> (w408:enum16{"非严格判断", "严格判断", "不判断"})
        n209 = global read "断电保存全局.vi" "数据发送通道"() -> (w404:enum16{"TCP", "VISA"})
        n210 = global read "断电保存全局.vi" "每周自动重发"() -> (w410:bool)
        n211 = global read "断电保存全局.vi" "数据发送协议"() -> (w405:enum16{"2005-212协议", "2017-212协议"})
        n212 = global read "断电保存全局.vi" "数据组合发送"() -> (w406:bool)
        n213 = global read "断电保存全局.vi" "VISA resource name"() -> (w412:refnum<visa-resource-name>)
        n214 = global read "断电保存全局.vi" "暂停上传"() -> (w400:bool)
        n215 = local write "baud rate"(w411) -> ()
        n216 = local write "2011发送"(w407) -> ()
        n217 = local write "重发时间"(w402) -> ()
        n218 = local write "站点设备"(w417) -> ()
        n219 = local write "站点名称"(w418) -> ()
        n220 = local write "重发日期"(w409) -> ()
        n221 = local write "判断数据反馈"(w408) -> ()
        n222 = local write "数据发送通道"(w404) -> ()
        n223 = local write "每周自动重发"(w410) -> ()
        n224 = local write "系统编码选择框"(w403) -> ()
        n225 = local write "数据发送协议"(w405) -> ()
        n226 = local write "数据组合发送"(w406) -> ()
        n227 = local write "暂停上传"(w400) -> ()
        n228 = local write "VISA resource name"(w412) -> ()
        n229 = local read "updateconfiguration"() -> (w401:T2)
        n230 = global read "全局1.vi" "软件自动重启"() -> (→"数据库打开失败次数":dbl)
        n231 = global write "update全局.vi" "updateconfiguration"(w401) -> ()
      }
    }
    n232 = flat-sequence {
      frame #0 {
        # "界面控件显示"
        n233 = global read "全局1.vi" "核查数据上传"() -> (→"核查数据上传":bool)
        n234 = global read "全局 数据发送重叠.vi" "掉线指示灯"() -> (→"掉线指示":bool)
        n235 = global read "全局1.vi" "实时小时数据上传"() -> (→"实时小时数据上传":bool)
        n236 = global read "全局1.vi" "系统状态"() -> (w343:bool)
        n237 = global read "全局1.vi" "运行模式"() -> (w344:bool)
        n238 = global read "全局1.vi" "测量周期"() -> (w345:bool)
        n239 = global read "全局1.vi" "超标留样"() -> (w346:bool)
        n240 = global read "全局1.vi" "与工控软件通信"() -> (→"与工控通信指示灯":bool)
        n241 = global read "全局1.vi" "反控数据"() -> (→"反控数据发送":bool)
        n242 = global read "全局1.vi" "发送报文显示"() -> (→"发送报文显示":string)
        n243 = global read "全局1.vi" "数据发送起始时间"() -> (w340:timestamp)
        n244 = global read "全局1.vi" "通讯包字符串"() -> (w357:string)
        n245 = global read "全局1.vi" "读取报文显示"() -> (→"读取报文显示":string)
        n246 = local read "数据发送通道"() -> (w351:enum16{"TCP", "VISA"})
        n247 = local read "数据发送协议"() -> (w365:enum16{"2005-212协议", "2017-212协议"})
        n248 = local read "数据发送通道"() -> (w376:enum16{"TCP", "VISA"})
        n249 = global read "全局 数据发送重叠.vi" "数据接收超时指示灯"() -> (→"数据接收超时指示灯":bool)
        n250 = Compound Arithmetic op=OR ("复合运算")(w343, w344, w345, w346) -> (→"系统状态改变":bool)
        n251 = case shown="\"VISA\"" w351 {
          frame "TCP", Default {
            w383 = TRUE ("可见")
            w384 = FALSE ("可见")
            n252 = property on="IP" class="Str"("Visible"=w383) -> ()  [unwired: 2 in, 2 out]
            n253 = property on="PORT" class="Str"("Visible"=w383) -> ()  [unwired: 2 in, 2 out]
            n254 = property on="VISA resource name" class="VISAName"("Visible"=w384) -> ()  [unwired: 2 in, 2 out]
            n255 = property on="baud rate" class="DigNum (严格)"("Visible"=w384) -> ()  [unwired: 2 in, 2 out]
          }
          frame "VISA" {
            w385 = FALSE ("可见")
            w386 = TRUE ("可见")
            n256 = property on="IP" class="Str"("Visible"=w385) -> ()  [unwired: 2 in, 2 out]
            n257 = property on="PORT" class="Str"("Visible"=w385) -> ()  [unwired: 2 in, 2 out]
            n258 = property on="VISA resource name" class="VISAName"("Visible"=w386) -> ()  [unwired: 2 in, 2 out]
            n259 = property on="baud rate" class="DigNum (严格)"("Visible"=w386) -> ()  [unwired: 2 in, 2 out]
          }
        }
        n260 = case shown="\"VISA\"" w376 {
          tunnel: [w395 w398] -> w373
          tunnel: [w394 w396] -> w370
          frame "TCP", Default {
            n261 = local read "PORT"() -> (w394:string)
            n262 = local read "IP"() -> (w395:string)
          }
          frame "VISA" {
            n263 = local read "VISA resource name"() -> (w398:refnum<visa-resource-name>)
            n264 = local read "baud rate"() -> (w397:u32)
            n265 = Number To Decimal String(number=w397) -> (decimal integer string=w396:string)  [unwired: 1 in]
          }
        }
        n266 = feedback #1(w357) -> (w358:string)
        n267 = feedback-in #1(w357) -> ()
        n268 = case shown="\"2017-212协议\"" w365 {
          tunnel: ["32" ("设备编码MN") w389] -> w364
          frame "2005-212协议", Default {
          }
          frame "2017-212协议" {
            n269 = global read "断电保存全局.vi" "系统编码选择框"() -> (w390:string)
            n270 = case shown="\"污水排放过程监测\"" w390 {
              tunnel: ["52" ("设备编码MN") "32" ("设备编码MN") "21" ("设备编码MN")] -> w389
              frame "污水排放过程监测" {
              }
              frame "地表水体污染源" {
              }
              frame "地表水质量监测", Default {
              }
            }
          }
        }
        n271 = Not Equal?(x=w357, y=w358) -> (x != y?=w356:bool)
        n272 = Get Date/Time In Seconds() -> (seconds since 1Jan1904=w366:timestamp)
        n273 = feedback #2(w340) -> (w342:timestamp)
        n274 = feedback-in #2(w340) -> ()
        n275 = case shown="真" w356 {
          tunnel: w357 -> [_ w387]
          frame False {
          }
          frame True {
            n276 = global write "全局1.vi" "发送报文显示"(w387) -> ()
          }
        }
        n277 = global read "断电保存全局.vi" "配置表格"() -> (w338:string[][])
        n278 = Format Date/Time String(time format string (%c)="%Y/%m/%d %H:%M:%S" ("时间格式字符串(%c)"), seconds (now)=w366) -> (date/time string=→"系统时间":string)  [unwired: 1 in]
        n279 = Select(t=T16."Enabled" ("禁用"), s="更改起始时间", f=T16."Disabled and Grayed Out" ("禁用")) -> (s? t:f=w352:T16)
        n280 = Not Equal?(x=w340, y=w342) -> (x != y?=w341:bool)
        n281 = property on="数据发送起始时间" class="AbsTime (严格)"("DisabledEnum"=w352) -> ()  [unwired: 2 in, 2 out]
        n282 = property on="确定更改起始时间" class="Bool"("DisabledEnum"=w352) -> ()  [unwired: 2 in, 2 out]
        n283 = case shown="真" w341 {
          tunnel: w340 -> [_ w382]
          frame False {
          }
          frame True {
            n284 = local write "数据发送起始时间"(w382) -> ()
          }
        }
        n285 = Index Array(array=w338, index (col) #1=1 ("禁用的索引 (列)"), index (col) #2=2 ("索引 (列)"), index (col) #3=3 ("索引 (列)")) -> (element #1=w336:string[], element #2=w330:string[], element #3=w332:string[])  [unwired: 3 in]
        n286 = for {
          tunnel: w332 -> [w381] mode=indexing
          tunnel: [w379] -> w331 mode=indexing
          n287 = Equal?(x=w381, y="启用") -> (x = y?=w379:bool)
        }
        n288 = for {
          tunnel: w330 -> [w378] mode=indexing
          tunnel: [w377] -> w329 mode=indexing
          n289 = Fract/Exp String To Number(string=w378) -> (number=w377:dbl)  [unwired: 3 in, 1 out]
        }
        n290 = Array To Cluster(array=w336) -> (cluster=w339:T17)
        n291 = local read "站点名称"() -> (w372:string)
        n292 = local read "站点设备"() -> (w371:string)
        n293 = global write "断电保存全局.vi" "因子编码簇"(w339) -> ()
        n294 = local read "MN"() -> (w369:string)
        n295 = Array To Cluster(array=w329) -> (cluster=w333:T18)
        n296 = global write "断电保存全局.vi" "参数启用数组"(w331) -> ()
        n297 = local read "PW"() -> (w368:string)
        n298 = global write "断电保存全局.vi" "参数系数簇"(w333) -> ()
        n299 = global write "全局1.vi" "系统编码ST"(w364) -> ()
        n300 = Bundle By Name(cluster=T6 {"站点"="", "设备"="", "IP"="", "PORT"="", "MN"="", "PW"=""} ("配置信息"), "站点"=w372, "设备"=w371, "IP"=w373, "PORT"=w370, "MN"=w369, "PW"=w368) -> (→"配置信息":T6)
      }
    }
    n301 = Wait (ms)(milliseconds to wait=u32 1000 ("等待时间（毫秒）")) -> ()  [unwired: 1 out]
  }
  n302 = while {
    stop <- FALSE stop-if-true
    n303 = event shown="[10] \"更新\": 值改变" {
      selector: _ -> [_ _ _ _ _ _ _ _ _ _ _ _ _]
      dyn-events: _ -> [_ _ _ _ _ _ _ _ _ _ _ _ _]
      timeout: _ -> [_ _ _ _ _ _ _ _ _ _ _ _ _]
      event Timeout {
        n304 = event-data() -> ()  [unwired: 1 in, 3 out]
      }
      event Panel Close? {
        n305 = event-data() -> ()  [unwired: 1 in, 3 out]
        n306 = Two Button Dialog(message="请确认是否关闭，关闭后数据将停止上传！" ("消息")) -> (T button?=w422:bool)  [unwired: 2 in]
        n307 = Not(x=w422) -> (.not. x?=w421:bool)
        n308 = event-data("Discard?"=w421) -> ()  [unwired: 1 in, 1 out]
      }
      event "站点名称", "站点设备", "IP", "PORT", "MN", "PW", "VISA resource name", "baud rate", "系统编码选择框", "每周自动重发", "重发日期", "重发时间", "暂停上传": Value Change {
        n309 = event-data() -> ("CtlRef"=w424:refnum<vi>)  [unwired: 1 in, 5 out]
        n310 = flat-sequence {
          tunnel: w424 -> [w426]
          tunnel: [w425] -> w423
          tunnel: w423 -> [w440]
          frame #0 {
            n311 = global write "断电保存全局.vi" "PW"("PW") -> ()
            n312 = global write "断电保存全局.vi" "站点名称"("站点名称") -> ()
            n313 = global write "断电保存全局.vi" "MN"("MN") -> ()
            n314 = global write "断电保存全局.vi" "PORT"("PORT") -> ()
            n315 = global write "断电保存全局.vi" "IP"("IP") -> ()
            n316 = global write "断电保存全局.vi" "重发日期"("重发日期") -> ()
            n317 = global write "断电保存全局.vi" "重发时间"("重发时间") -> ()
            n318 = global write "断电保存全局.vi" "站点设备"("站点设备") -> ()
            n319 = global write "断电保存全局.vi" "baud rate"("baud rate") -> ()
            n320 = global write "断电保存全局.vi" "系统编码选择框"("系统编码选择框") -> ()
            n321 = global write "断电保存全局.vi" "每周自动重发"("每周自动重发") -> ()
            n322 = global write "断电保存全局.vi" "暂停上传"("暂停上传") -> ()
            n323 = global write "断电保存全局.vi" "VISA resource name"("VISA resource name") -> ()
            n324 = property class="Ctl"(reference=w426) -> ("Caption.Text"=w425:string)  [unwired: 1 in, 2 out]
          }
          frame #1 {
            n325 = case shown="\"IP\", \"PORT\"" w440 {
              frame "假", Default {
              }
              frame "IP", "PORT" {
                n326 = call "通信状态入队列.vi"("枚举"=enum16{"打开连接", "发送数据", "读取数据", "数据处理", "关闭连接"}."关闭连接") -> ()  [unwired: 10 in, 1 out]
              }
            }
            n327 = call "配置文件断电保存(子VI).vi"() -> ()  [unwired: 12 in]
          }
        }
      }
      event "数据发送通道", "数据发送协议", "数据组合发送", "2011发送": Value Change {
        n328 = event-data() -> ("CtlRef"=w445:refnum<vi>, "OldVal"=w443:variant, "NewVal"=w442:variant)  [unwired: 1 in, 3 out]
        n329 = property class="Ctl"(reference=w445) -> ("Label.Text"=w444:string)  [unwired: 1 in, 2 out]
        n330 = case shown="\"判断数据反馈\"" w444 {
          tunnel: w443 -> [_ w449 w472 w481 w504 w527 w548]
          tunnel: w442 -> [_ w446 w469 w478 w501 w524 w547]
          frame "假", Default {
          }
          frame "数据发送通道" {
            n331 = Variant To Data(type=enum16{"TCP", "VISA"}."TCP" ("数据发送通道"), Variant=w446) -> (data=w447:enum16{"TCP", "VISA"})  [unwired: 1 in, 1 out]
            n332 = global write "断电保存全局.vi" "数据发送通道"(w447) -> ()
            n333 = Two Button Dialog(message="TCP通过网络发送数据，VISA通过串口发送数据，确定更改数据发送通道吗？" ("消息")) -> (T button?=w450:bool)  [unwired: 2 in]
            n334 = case shown="假" w450 {
              tunnel: w449 -> [w453 _]
              frame False {
                n335 = Variant To Data(type=enum16{"TCP", "VISA"}."TCP" ("数据发送通道"), Variant=w453) -> (data=w452:enum16{"TCP", "VISA"})  [unwired: 1 in, 1 out]
                n336 = global write "断电保存全局.vi" "数据发送通道"(w452) -> ()
              }
              frame True {
                n337 = flat-sequence {
                  frame #0 {
                  }
                  frame #1 {
                    n338 = call <vilib>:"Application Directory.vi"() -> ("Application Directory"=w455:path)
                    n339 = Build Path(base path=w455, name or relative path="data\\sys.ini" ("名称或相对路径")) -> (appended path=w457:path)
                    n340 = call <vilib>:"Open Config Data.vi"("configuration file path"=w457) -> ("error out"=w461:errorcluster, "refnum"=w458:T13)  [unwired: 8 in, 1 out]
                    n341 = vi-ref "断电保存全局.vi"() -> (w459:refnum<vi>)
                    n342 = call <userlib>:"Write Panel to INI__ogtk.vi"("error in (no error)"=w461, "VI ref"=w459, "refnum"=w458) -> ("error out"=w462:errorcluster, "refnum out"=w460:T13)  [unwired: 7 in]
                    n343 = call <vilib>:"Close Config Data.vi"("error in (no error)"=w462, "refnum"=w460) -> ("error out"=w467:errorcluster, "file path"=w468:path)  [unwired: 8 in]
                    n344 = Open/Create/Replace File(file path (use dialog)=w468, error in=w467) -> (refnum out=w464:refnum<file>, error out=w463:errorcluster)  [unwired: 4 in, 1 out]
                    n345 = Flush File(refnum=w464, error in=w463) -> (refnum out=w465:refnum<file>, error out=w466:errorcluster)
                    n346 = Close File(refnum=w465, error in=w466) -> ()  [unwired: 2 out]
                  }
                }
              }
            }
          }
          frame "数据发送协议" {
            n347 = Variant To Data(type=enum16{"2005-212协议", "2017-212协议"}."2017-212协议" ("数据"), Variant=w469) -> (data=w470:enum16{"2005-212协议", "2017-212协议"})  [unwired: 1 in, 1 out]
            n348 = global write "断电保存全局.vi" "数据发送协议"(w470) -> ()
            n349 = Two Button Dialog(message="2005对应旧版通信协议，2017对应最新版协议，对应协议因子编码会不同，\n更改可能导致数据不能被平台识别，确定更改数据发送协议吗？" ("消息")) -> (T button?=w473:bool)  [unwired: 2 in]
            n350 = case shown="真" w473 {
              tunnel: w472 -> [w477 _]
              frame False {
                n351 = Variant To Data(type=enum16{"2005-212协议", "2017-212协议"}."2017-212协议" ("数据"), Variant=w477) -> (data=w475:enum16{"2005-212协议", "2017-212协议"})  [unwired: 1 in, 1 out]
                n352 = global write "断电保存全局.vi" "数据发送协议"(w475) -> ()
              }
              frame True {
                n353 = call "配置文件断电保存(子VI).vi"() -> ()  [unwired: 12 in]
              }
            }
          }
          frame "数据组合发送" {
            n354 = Variant To Data(type=FALSE, Variant=w478) -> (data=w479:bool)  [unwired: 1 in, 1 out]
            n355 = global write "断电保存全局.vi" "数据组合发送"(w479) -> ()
            n356 = Two Button Dialog(message="勾选数据组合发送功能表示所有参数打包整点同时上传、则只能整点发送延时较高，\n不勾选则表示单参数分别上传、则实时性较好，确定更改数据组合发送功能吗？" ("消息")) -> (T button?=w482:bool)  [unwired: 2 in]
            n357 = case shown="真" w482 {
              tunnel: w481 -> [w485 _]
              frame False {
                n358 = Variant To Data(type=FALSE, Variant=w485) -> (data=w484:bool)  [unwired: 1 in, 1 out]
                n359 = global write "断电保存全局.vi" "数据组合发送"(w484) -> ()
              }
              frame True {
                n360 = flat-sequence {
                  frame #0 {
                  }
                  frame #1 {
                    n361 = call <vilib>:"Application Directory.vi"() -> ("Application Directory"=w487:path)
                    n362 = Build Path(base path=w487, name or relative path="data\\sys.ini" ("名称或相对路径")) -> (appended path=w489:path)
                    n363 = call <vilib>:"Open Config Data.vi"("configuration file path"=w489) -> ("error out"=w493:errorcluster, "refnum"=w490:T13)  [unwired: 8 in, 1 out]
                    n364 = vi-ref "断电保存全局.vi"() -> (w491:refnum<vi>)
                    n365 = call <userlib>:"Write Panel to INI__ogtk.vi"("error in (no error)"=w493, "VI ref"=w491, "refnum"=w490) -> ("error out"=w494:errorcluster, "refnum out"=w492:T13)  [unwired: 7 in]
                    n366 = call <vilib>:"Close Config Data.vi"("error in (no error)"=w494, "refnum"=w492) -> ("error out"=w499:errorcluster, "file path"=w500:path)  [unwired: 8 in]
                    n367 = Open/Create/Replace File(file path (use dialog)=w500, error in=w499) -> (refnum out=w496:refnum<file>, error out=w495:errorcluster)  [unwired: 4 in, 1 out]
                    n368 = Flush File(refnum=w496, error in=w495) -> (refnum out=w497:refnum<file>, error out=w498:errorcluster)
                    n369 = Close File(refnum=w497, error in=w498) -> ()  [unwired: 2 out]
                  }
                }
              }
            }
          }
          frame "2011发送" {
            n370 = Variant To Data(type=FALSE, Variant=w501) -> (data=w502:bool)  [unwired: 1 in, 1 out]
            n371 = global write "断电保存全局.vi" "2011发送"(w502) -> ()
            n372 = Two Button Dialog(message="2011表示实时数据上传，一般情况需要勾选，确定更改2011实时数据发送功能吗？" ("消息")) -> (T button?=w505:bool)  [unwired: 2 in]
            n373 = case shown="真" w505 {
              tunnel: w504 -> [w508 _]
              frame False {
                n374 = Variant To Data(type=FALSE, Variant=w508) -> (data=w507:bool)  [unwired: 1 in, 1 out]
                n375 = global write "断电保存全局.vi" "2011发送"(w507) -> ()
              }
              frame True {
                n376 = flat-sequence {
                  frame #0 {
                  }
                  frame #1 {
                    n377 = call <vilib>:"Application Directory.vi"() -> ("Application Directory"=w510:path)
                    n378 = Build Path(base path=w510, name or relative path="data\\sys.ini" ("名称或相对路径")) -> (appended path=w512:path)
                    n379 = call <vilib>:"Open Config Data.vi"("configuration file path"=w512) -> ("error out"=w516:errorcluster, "refnum"=w513:T13)  [unwired: 8 in, 1 out]
                    n380 = vi-ref "断电保存全局.vi"() -> (w514:refnum<vi>)
                    n381 = call <userlib>:"Write Panel to INI__ogtk.vi"("error in (no error)"=w516, "VI ref"=w514, "refnum"=w513) -> ("error out"=w517:errorcluster, "refnum out"=w515:T13)  [unwired: 7 in]
                    n382 = call <vilib>:"Close Config Data.vi"("error in (no error)"=w517, "refnum"=w515) -> ("error out"=w522:errorcluster, "file path"=w523:path)  [unwired: 8 in]
                    n383 = Open/Create/Replace File(file path (use dialog)=w523, error in=w522) -> (refnum out=w519:refnum<file>, error out=w518:errorcluster)  [unwired: 4 in, 1 out]
                    n384 = Flush File(refnum=w519, error in=w518) -> (refnum out=w520:refnum<file>, error out=w521:errorcluster)
                    n385 = Close File(refnum=w520, error in=w521) -> ()  [unwired: 2 out]
                  }
                }
              }
            }
          }
          frame "日志、参数发送" {
            n386 = Variant To Data(type=FALSE, Variant=w524) -> (data=w525:bool)  [unwired: 1 in, 1 out]
            n387 = global write "断电保存全局.vi" "日志、参数发送"(w525) -> ()
            n388 = Two Button Dialog(message="选择是否需要仪器日志、状态和告警信息上传，一般情况需要勾选，确定更改日志、参数发送功能吗？" ("消息")) -> (T button?=w528:bool)  [unwired: 2 in]
            n389 = case shown="假" w528 {
              tunnel: w527 -> [w531 _]
              frame False {
                n390 = Variant To Data(type=FALSE, Variant=w531) -> (data=w530:bool)  [unwired: 1 in, 1 out]
                n391 = global write "断电保存全局.vi" "日志、参数发送"(w530) -> ()
              }
              frame True {
                n392 = flat-sequence {
                  frame #0 {
                  }
                  frame #1 {
                    n393 = call <vilib>:"Application Directory.vi"() -> ("Application Directory"=w533:path)
                    n394 = Build Path(base path=w533, name or relative path="data\\sys.ini" ("名称或相对路径")) -> (appended path=w535:path)
                    n395 = call <vilib>:"Open Config Data.vi"("configuration file path"=w535) -> ("error out"=w539:errorcluster, "refnum"=w536:T13)  [unwired: 8 in, 1 out]
                    n396 = vi-ref "断电保存全局.vi"() -> (w537:refnum<vi>)
                    n397 = call <userlib>:"Write Panel to INI__ogtk.vi"("error in (no error)"=w539, "VI ref"=w537, "refnum"=w536) -> ("error out"=w540:errorcluster, "refnum out"=w538:T13)  [unwired: 7 in]
                    n398 = call <vilib>:"Close Config Data.vi"("error in (no error)"=w540, "refnum"=w538) -> ("error out"=w545:errorcluster, "file path"=w546:path)  [unwired: 8 in]
                    n399 = Open/Create/Replace File(file path (use dialog)=w546, error in=w545) -> (refnum out=w542:refnum<file>, error out=w541:errorcluster)  [unwired: 4 in, 1 out]
                    n400 = Flush File(refnum=w542, error in=w541) -> (refnum out=w543:refnum<file>, error out=w544:errorcluster)
                    n401 = Close File(refnum=w543, error in=w544) -> ()  [unwired: 2 out]
                  }
                }
              }
            }
          }
          frame "判断数据反馈" {
            n402 = Two Button Dialog(message="判断数据反馈是针对平台能有反馈的情况，\n1.严格判断反馈-收不到反馈一直重发\n2.非严格判断-重发5次后跳过该数据\n3.不判断反馈针对平台没有反馈的情况\n确定更改判断数据反馈功能吗？" ("消息")) -> (T button?=w549:bool)  [unwired: 2 in]
            n403 = case shown="假" w549 {
              tunnel: w548 -> [_ _]
              tunnel: w547 -> [w552 w554]
              frame False {
                n404 = Variant To Data(type=enum16{"非严格判断", "严格判断", "不判断"}."非严格判断" ("判断数据反馈"), Variant=w552) -> (data=w551:enum16{"非严格判断", "严格判断", "不判断"})  [unwired: 1 in, 1 out]
                n405 = local write "判断数据反馈"(w551) -> ()
              }
              frame True {
                n406 = flat-sequence {
                  tunnel: w554 -> [w555]
                  frame #0 {
                    n407 = Variant To Data(type=enum16{"非严格判断", "严格判断", "不判断"}."非严格判断" ("判断数据反馈"), Variant=w555) -> (data=w557:enum16{"非严格判断", "严格判断", "不判断"})  [unwired: 1 in, 1 out]
                    n408 = global write "断电保存全局.vi" "判断数据反馈"(w557) -> ()
                  }
                  frame #1 {
                    n409 = call <vilib>:"Application Directory.vi"() -> ("Application Directory"=w558:path)
                    n410 = Build Path(base path=w558, name or relative path="data\\sys.ini" ("名称或相对路径")) -> (appended path=w560:path)
                    n411 = call <vilib>:"Open Config Data.vi"("configuration file path"=w560) -> ("error out"=w564:errorcluster, "refnum"=w561:T13)  [unwired: 8 in, 1 out]
                    n412 = vi-ref "断电保存全局.vi"() -> (w562:refnum<vi>)
                    n413 = call <userlib>:"Write Panel to INI__ogtk.vi"("error in (no error)"=w564, "VI ref"=w562, "refnum"=w561) -> ("error out"=w565:errorcluster, "refnum out"=w563:T13)  [unwired: 7 in]
                    n414 = call <vilib>:"Close Config Data.vi"("error in (no error)"=w565, "refnum"=w563) -> ("error out"=w570:errorcluster, "file path"=w571:path)  [unwired: 8 in]
                    n415 = Open/Create/Replace File(file path (use dialog)=w571, error in=w570) -> (refnum out=w567:refnum<file>, error out=w566:errorcluster)  [unwired: 4 in, 1 out]
                    n416 = Flush File(refnum=w567, error in=w566) -> (refnum out=w568:refnum<file>, error out=w569:errorcluster)
                    n417 = Close File(refnum=w568, error in=w569) -> ()  [unwired: 2 out]
                  }
                }
              }
            }
          }
        }
      }
      event "确定": Value Change {
        n418 = event-data() -> ()  [unwired: 1 in, 6 out]
        n419 = call "通信状态入队列.vi"("枚举"=enum16{"打开连接", "发送数据", "读取数据", "数据处理", "关闭连接"}."关闭连接") -> ()  [unwired: 10 in, 1 out]
      }
      event "配置表": Value Change {
        n420 = event-data() -> ()  [unwired: 1 in, 6 out]
        n421 = call "参数配置表.vi"() -> ()  [unwired: 12 in]
      }
      event "参数配置": Value Change {
        n422 = event-data() -> ()  [unwired: 1 in, 6 out]
        n423 = property on="窗格" class="Pane"("Origin"=T10 {"Horizontal"=0, "Vertical"=1000} ("原点")) -> ()  [unwired: 2 in, 2 out]
        n424 = call <vilib>:"Application Directory.vi"() -> ("Application Directory"=w574:path)
        n425 = call "查询启动项.vi"("启动文件路径"=w574) -> ("包含启动项"=w573:bool)  [unwired: 9 in, 1 out]
        n426 = local write "开机启动"(w573) -> ()
      }
      event "返回": Value Change {
        n427 = event-data() -> ()  [unwired: 1 in, 6 out]
        n428 = property on="窗格" class="Pane"("Origin"=T10 {"Horizontal"=0, "Vertical"=0} ("原点")) -> ()  [unwired: 2 in, 2 out]
      }
      event "确定更改起始时间": Value Change {
        n429 = event-data() -> ()  [unwired: 1 in, 6 out]
        n430 = local write "更改起始时间"(FALSE ("更改起始时间")) -> ()
        n431 = Two Button Dialog(message="确定以当前设置时间作为数据索引起始时间？" ("消息")) -> (T button?=w577:bool)  [unwired: 2 in]
        n432 = case shown="真" w577 {
          frame False {
          }
          frame True {
            n433 = global write "断电保存全局.vi" "数据重发"(TRUE ("数据重发")) -> ()
            n434 = Format Date/Time String(time format string (%c)="%Y/%m/%d %H:%M:%S" ("时间格式字符串(%c)"), seconds (now)="数据发送起始时间") -> (date/time string=w580:string)  [unwired: 1 in]
            n435 = global write "断电保存全局.vi" "数据重发时间戳"(w580) -> ()
            n436 = Initialize Array(w580, 31 ("维数大小")) -> (w585:string[])
            n437 = Initialize Array(w580, 13 ("维数大小")) -> (w581:string[])
            n438 = Array To Cluster(array=w585) -> (cluster=w584:T15)
            n439 = Array To Cluster(array=w581) -> (cluster=w582:T19)
            n440 = global write "全局 时间2.vi" "仪器参数索引"(w582) -> ()
            n441 = global write "全局 水样时间.vi" "水样数据索引"(w584) -> ()
            n442 = global read "断电保存全局.vi" "数据组合发送"() -> (w589:bool)
            n443 = case shown="假" w589 {
              tunnel: w580 -> [w591 _]
              frame False {
                n444 = global write "全局 时间2.vi" "标样核查索引起始时间"(w591) -> ()
                n445 = global write "全局 时间2.vi" "加标回收索引起始时间"(w591) -> ()
                n446 = global write "全局 时间2.vi" "跨度核查索引起始时间"(w591) -> ()
                n447 = global write "全局 时间2.vi" "零点核查索引起始时间"(w591) -> ()
                n448 = Initialize Array(w591, 8 ("维数大小")) -> (w600:string[])
                n449 = Initialize Array(w591, 15 ("维数大小")) -> (w595:string[])
                n450 = Array To Cluster(array=w600) -> (cluster=w599:T20)
                n451 = Array To Cluster(array=w595) -> (cluster=w596:T21)
                n452 = global write "全局 时间2.vi" "零点核查索引"(w599) -> ()
                n453 = global write "全局 时间2.vi" "跨度核查索引"(w599) -> ()
                n454 = global write "全局 时间2.vi" "标样核查索引"(w596) -> ()
                n455 = global write "全局 时间2.vi" "集成干预索引"(w596) -> ()
                n456 = Initialize Array(w591, 5 ("维数大小")) -> (w592:string[])
                n457 = Array To Cluster(array=w592) -> (cluster=w593:T22)
                n458 = global write "全局 时间2.vi" "加标回收索引"(w593) -> ()
                n459 = global write "全局 时间2.vi" "平行样索引"(w593) -> ()
              }
              frame True {
              }
            }
          }
        }
      }
      event "开机启动": Value Change {
        n460 = event-data() -> ("CtlRef"=w602:refnum<vi>, "OldVal"=w601:bool, "NewVal"=w603:bool)  [unwired: 1 in, 3 out]
        n461 = case shown="真" w603 {
          tunnel: w602 -> [w605 w618]
          tunnel: w601 -> [w604 w617]
          frame False {
            n462 = Two Button Dialog(message="是否删除开机启动？" ("消息"), 1:"否" ("F按钮名称（“取消”）"), 2:"是" ("T按钮名称（“确定”）")) -> (T button?=w606:bool)
            n463 = case shown="假" w606 {
              tunnel: w605 -> [w611 _]
              tunnel: w604 -> [w610 _]
              frame False {
                n464 = property class="Bool (严格)"(reference=w611, "Value"=w610) -> ()  [unwired: 1 in, 2 out]
              }
              frame True {
                n465 = call <vilib>:"Application Directory.vi"() -> ("Application Directory"=w613:path)
                n466 = call "删除启动项.vi"("启动文件路径"=w613) -> ("删除标记"=w612:bool)  [unwired: 9 in, 1 out]
                n467 = case shown="假" w612 {
                  tunnel: ["删除开机启动失败" ("T按钮名称（“确定”）") "删除开机启动成功" ("T按钮名称（“确定”）")] -> w614
                  frame False {
                  }
                  frame True {
                  }
                }
                n468 = One Button Dialog(message=w614) -> ()  [unwired: 1 in, 1 out]
              }
            }
          }
          frame True {
            n469 = Two Button Dialog(message="是否添加开机启动？" ("消息"), 1:"否" ("F按钮名称（“取消”）"), 2:"是" ("T按钮名称（“确定”）")) -> (T button?=w619:bool)
            n470 = case shown="真" w619 {
              tunnel: w618 -> [w624 _]
              tunnel: w617 -> [w623 _]
              frame False {
                n471 = property class="Bool (严格)"(reference=w624, "Value"=w623) -> ()  [unwired: 1 in, 2 out]
              }
              frame True {
                n472 = call <vilib>:"Application Directory.vi"() -> ("Application Directory"=w627:path)
                n473 = call "添加启动项.vi"("启动文件路径"=w627) -> ("添加成功标记"=w626:bool)  [unwired: 9 in, 1 out]
                n474 = case shown="真" w626 {
                  tunnel: ["添加开机启动失败" ("T按钮名称（“确定”）") "添加开机启动成功" ("T按钮名称（“确定”）")] -> w625
                  frame False {
                  }
                  frame True {
                  }
                }
                n475 = One Button Dialog(message=w625) -> ()  [unwired: 1 in, 1 out]
              }
            }
          }
        }
      }
      event "更新": Value Change {
        n476 = event-data() -> ()  [unwired: 1 in, 6 out]
        n477 = call "自定义双按钮对话框.vi"("消息"="选择是否从服务器获取最新版本信息？") -> ("输出"=w630:bool)  [unwired: 10 in]
        n478 = case shown="真" w630 {
          frame False {
          }
          frame True {
            w638 = T9 2 items=["两端", "字符串首端", "字符串末端"] ("location (both)")
            w634 = "/" ("分隔符(Tab)")
            # "获取最新版本"
            n479 = local read "updateconfiguration"() -> (w647:T2)
            n480 = Unbundle By Name(w647) -> ("主机"=w646:string, "用户"=w635:string, "密码"=w645:string, "远程路径"=w643:string)
            n481 = Spreadsheet String To Array(delimiter (Tab)="\\" ("分隔符(Tab)"), format string="" ("格式字符串"), spreadsheet string=w643, array type (2D Dbl)=string[] []) -> (array=w640:string[])
            n482 = Array To Spreadsheet String(delimiter (Tab)=w634, array=w640, 3:"%s" ("格式字符串")) -> (spreadsheet string=w633:string)
            n483 = Concatenate Strings(w634, w633) -> (w632:string)
            n484 = call <vilib>:"Trim Whitespace.vi"("string"=w632, "location (both)"=w638) -> ("trimmed string"=w637:string)
            n485 = Bundle By Name(cluster=T7 {"host"="27.154.58.30", "port"=8020, "user"="std", "password"="std23506", "远端地址"="/微站/室外总磷总氮高压过滤无主板新电路板/一体化微型水质监测站.exe"} ("服务器信息"), "host"=w646, "port"=u16 8020, "user"=w635, "password"=w645, "远端地址"=w637) -> (w648:T7)
            n486 = call "Update.vi"("服务器信息"=w648) -> ()  [unwired: 11 in]
          }
        }
      }
      event "updateconfiguration": Value Change {
        n487 = event-data() -> ("NewVal"=w657:T2)  [unwired: 1 in, 5 out]
        n488 = call <vilib>:"Application Directory.vi"() -> ("Application Directory"=w661:path)
        n489 = Build Array("主机" ("section"), "用户" ("section"), "密码" ("key"), "远程路径" ("key"), "下载文件名" ("key"), "软件版本" ("key")) -> (w650:string[])
        n490 = Build Path(base path=w661, name or relative path="update\\data\\set.ini" ("名称或相对路径")) -> (appended path=w659:path)
        n491 = call "配置文件write.vi"("updateconfiguration"=w657, "configuration file path"=w659, "键数组"=w650, "段"="应用程序交互" ("section")) -> ("error out"=w658:errorcluster)  [unwired: 7 in]
        n492 = call <vilib>:"Clear Errors.vi"("error in (no error)"=w658) -> ()  [unwired: 5 in, 2 out]
      }
      event "IP", "PORT": Mouse Down {
        n493 = event-data() -> ("CtlRef"=w666:refnum<vi>)  [unwired: 1 in, 7 out]
        n494 = property class="Str"(reference=w666) -> (reference out=w664:refnum<vi>, "Value"=w665:string)  [unwired: 1 in, 1 out]
        n495 = call "IP键盘.vi"("OldNumber"=w665) -> ("NewNumber"=w663:string)
        n496 = property class="Str"(reference=w664, "Val(Sgnl)"=w663) -> ()  [unwired: 1 in, 2 out]
      }
    }
  }
  n497 = while {
    tunnel: w11 -> [w675]
    tunnel: w10 -> [w674]
    shift-right: [w670] -> _
    shift-left: errorcluster {"status"=FALSE, "code"=0, "source"=""} ("error out") -> [w669]
    stop <- FALSE stop-if-true
    # "写入数据出队列"
    n498 = Dequeue Element(queue=w675, timeout in ms (-1)=30000 ("超时毫秒(-1)"), error in (no error)=w674) -> (queue out=w668:refnum<queue>, element=w672:enum16{"打开连接", "发送数据", "读取数据", "数据处理", "关闭连接"}, timed out?=w671:bool, error out=w667:errorcluster)
    n499 = case shown="无错误" w669 {
      tunnel: w672 -> [w677 _]
      tunnel: w671 -> [w679 _]
      tunnel: [w683 w725] -> w670
      tunnel: w669 -> [w682 w729]
      tunnel: w668 -> [w681 w727]
      tunnel: w667 -> [w680 w726]
      frame No Error {
        n500 = case shown="真" w679 {
          tunnel: [w684 enum16{"打开连接", "发送数据", "读取数据", "数据处理", "关闭连接"}."发送数据" ("枚举")] -> w678
          tunnel: w677 -> [w684 _]
          frame False {
          }
          frame True {
          }
        }
        n501 = case shown="\"发送数据\", 默认" w678 {
          tunnel: w679 -> [_ w702 _ _ _]
          tunnel: [w687 w697 _ _ w718] -> w683
          tunnel: w682 -> [w689 w704 _ _ w719]
          tunnel: w681 -> [_ _ _ _ w720]
          tunnel: w680 -> [_ _ _ _ w717]
          frame "打开连接" {
            n502 = global read "断电保存全局.vi" "VISA resource name"() -> (w695:refnum<visa-resource-name>)
            n503 = global read "断电保存全局.vi" "数据发送通道"() -> (w692:enum16{"TCP", "VISA"})
            n504 = global read "断电保存全局.vi" "baud rate"() -> (w694:u32)
            n505 = global read "断电保存全局.vi" "PORT"() -> (w693:string)
            n506 = global read "断电保存全局.vi" "IP"() -> (w691:string)
            n507 = call "VISATCP组合选择发送.vi"("IP"=w691, "数据发送通道"=w692, "命令"="open", "PORT"=w693, "VISA resource name"=w695, "baud rate"=w694, "error in (no error)"=w689) -> ("错误输出"=w687:errorcluster)  [unwired: 5 in, 3 out]
            n508 = Unbundle By Name(w687) -> ("status"=w686:bool)  [unwired: 1 out]
            n509 = Not(x=w686) -> (.not. x?=w688:bool)
            n510 = global write "全局 数据发送重叠.vi" "掉线指示灯"(w686) -> ()
            n511 = local write "通信状态"(w688) -> ()
          }
          frame "发送数据", Default {
            n512 = case shown="真" w702 {
              tunnel: [w709 w711] -> w699
              tunnel: w704 -> [w708 w712]
              tunnel: [w708 w712] -> w703
              frame False {
                # "事件触发发送数据"
                n513 = global read "全局1.vi" "发送报文显示"() -> (w709:string)
              }
              frame True {
                # "30秒超时发送心跳包"
                n514 = local read "配置信息"() -> (w715:T6)
                n515 = Unbundle By Name(w715) -> ("MN"=w714:string, "PW"=w713:string)
                n516 = call "数据编码.vi"("table输入"="心跳包", "MN"=w714, "PW"=w713) -> ("通讯包字符串"=w711:string)  [unwired: 11 in, 1 out]
                n517 = global write "全局1.vi" "发送报文显示"(w711) -> ()
                n518 = Wait (ms)(milliseconds to wait=u32 500 ("等待时间（毫秒）")) -> ()  [unwired: 1 out]
              }
            }
            n519 = global read "断电保存全局.vi" "数据发送通道"() -> (w705:enum16{"TCP", "VISA"})
            n520 = Concatenate Strings("send:" ("字符串"), w699) -> (w698:string)
            n521 = call "VISATCP组合选择发送.vi"("数据发送通道"=w705, "命令"="write", "error in (no error)"=w703, "写入缓冲区"=w699) -> ("错误输出"=w697:errorcluster)  [unwired: 8 in, 3 out]
            n522 = Build Array(w698) -> (w701:string[])
            n523 = call "发送数据记录到文档(子VI).vi"("字符串"="报文记录", "数组"=w701) -> ()  [unwired: 8 in, 1 out]
            n524 = flat-sequence {
              tunnel: w697 -> [_]
              frame #0 {
                n525 = local write "心跳包"(FALSE ("心跳包")) -> ()
              }
            }
            "心跳包" <- w702
          }
          frame "读取数据" {
          }
          frame "数据处理" {
          }
          frame "关闭连接" {
            n526 = global read "断电保存全局.vi" "数据发送通道"() -> (w722:enum16{"TCP", "VISA"})
            n527 = Enqueue Element(queue=w720, element=enum16{"打开连接", "发送数据", "读取数据", "数据处理", "关闭连接"}."打开连接" ("枚举"), error in (no error)=w717) -> ()  [unwired: 1 in, 3 out]
            n528 = call "VISATCP组合选择发送.vi"("数据发送通道"=w722, "命令"="close", "error in (no error)"=w719) -> ("错误输出"=w723:errorcluster)  [unwired: 9 in, 3 out]
            n529 = call <vilib>:"Clear Errors.vi"("error in (no error)"=w723) -> ("error out"=w718:errorcluster)  [unwired: 5 in, 1 out]
          }
        }
      }
      frame Error {
        n530 = Unbundle By Name(w729) -> ("code"=w728:i32)
        n531 = case shown="0, 默认" w728 {
          tunnel: w727 -> [w736 w752 w764]
          tunnel: w726 -> [w735 w751 w763]
          tunnel: [w734 w749 w762] -> w725
          frame 0, Default {
            n532 = Flush Queue(queue=w736, error in (no error)=w735) -> (queue out=w738:refnum<queue>, error out=w739:errorcluster)  [unwired: 1 out]
            n533 = local read "状态信息"() -> (w733:T5)
            n534 = Unbundle By Name(w733) -> ("TCP服务端掉线计数"=w731:i32)
            n535 = Enqueue Element(queue=w738, element=enum16{"打开连接", "发送数据", "读取数据", "数据处理", "关闭连接"}."关闭连接" ("枚举"), error in (no error)=w739) -> (error out=w740:errorcluster)  [unwired: 1 in, 2 out]
            n536 = Increment(x=w731) -> (x+1=w732:i32)
            n537 = Bundle By Name(cluster=w733, "TCP服务端掉线计数"=w732) -> (w730:T5)
            n538 = local write "状态信息"(w730) -> ()
            n539 = call <vilib>:"Clear Errors.vi"("error in (no error)"=w740) -> ("error out"=w734:errorcluster)  [unwired: 5 in, 1 out]
          }
          frame 54, 63 {
            n540 = Flush Queue(queue=w752, error in (no error)=w751) -> (queue out=w754:refnum<queue>, error out=w755:errorcluster)  [unwired: 1 out]
            n541 = local read "状态信息"() -> (w744:T5)
            n542 = Unbundle By Name(w744) -> ("TCP服务端掉线计数"=w748:i32, "TCP掉线时间节点"=w741:string)
            n543 = Enqueue Element(queue=w754, element=enum16{"打开连接", "发送数据", "读取数据", "数据处理", "关闭连接"}."关闭连接" ("枚举"), error in (no error)=w755) -> (error out=w750:errorcluster)  [unwired: 1 in, 2 out]
            n544 = Less Or Equal?(x=w748, y=1) -> (x <= y?=w746:bool)
            n545 = case shown="真" w746 {
              tunnel: [w756 w757] -> w745
              tunnel: w741 -> [w756 _]
              frame False {
              }
              frame True {
                n546 = Get Date/Time In Seconds() -> (seconds since 1Jan1904=w758:timestamp)
                n547 = Format Date/Time String(time format string (%c)="%Y%m%d%H%M%S%3u" ("时间格式字符串(%c)"), seconds (now)=w758) -> (date/time string=w760:string)  [unwired: 1 in]
                n548 = call "格式时间字符串.vi"("字符串"=w760) -> ("连接的字符串"=w757:string)  [unwired: 10 in]
              }
            }
            n549 = Increment(x=w748) -> (x+1=w743:i32)
            n550 = call <vilib>:"Clear Errors.vi"("error in (no error)"=w750) -> ("error out"=w749:errorcluster)  [unwired: 5 in, 1 out]
            n551 = Bundle By Name(cluster=w744, "TCP服务端掉线计数"=w743, "TCP掉线时间节点"=w745) -> (w742:T5)
            n552 = local write "状态信息"(w742) -> ()
          }
          frame 56 {
            n553 = Flush Queue(queue=w764, error in (no error)=w763) -> (error out=w761:errorcluster)  [unwired: 2 out]
            n554 = call <vilib>:"Clear Errors.vi"("error in (no error)"=w761) -> ("error out"=w762:errorcluster)  [unwired: 5 in, 1 out]
          }
        }
      }
    }
  }
  n555 = while {
    tunnel: w8 -> [w777]
    tunnel: w7 -> [w776]
    shift-right: [w773] -> _
    shift-left: errorcluster {"status"=FALSE, "code"=0, "source"=""} ("error out") -> [w772]
    tunnel: w5 -> [w768]
    tunnel: w4 -> [w767]
    tunnel: w3 -> [w766]
    tunnel: w2 -> [w765]
    stop <- FALSE stop-if-true
    # "读取数据出队列处理"
    n556 = Dequeue Element(queue=w777, error in (no error)=w776) -> (queue out=w771:refnum<queue>, element=w774:enum16{"打开连接", "发送数据", "读取数据", "数据处理", "关闭连接"}, error out=w770:errorcluster)  [unwired: 1 in, 1 out]
    n557 = Wait (ms)(milliseconds to wait=u32 1000 ("等待时间（毫秒）")) -> ()  [unwired: 1 out]
    n558 = case shown="无错误" w772 {
      tunnel: w774 -> [w783 _]
      tunnel: [w790 w868] -> w773
      tunnel: w772 -> [w789 w872]
      tunnel: w771 -> [w788 w870]
      tunnel: w770 -> [w787 w869]
      tunnel: w768 -> [w781 _]
      tunnel: w767 -> [w780 _]
      tunnel: w766 -> [w779 _]
      tunnel: w765 -> [w778 _]
      frame No Error {
        n559 = case shown="\"读取数据\"" w783 {
          tunnel: [w797 _ w831 _ w863] -> w790
          tunnel: w789 -> [w796 _ w834 _ w864]
          tunnel: w788 -> [w794 _ w826 _ w861]
          tunnel: w787 -> [w793 _ w825 _ w860]
          tunnel: [w792 _ _ _ _] -> w784
          tunnel: w781 -> [_ _ w818 _ _]
          tunnel: w780 -> [_ _ w817 _ _]
          tunnel: w779 -> [_ _ w806 _ _]
          tunnel: w778 -> [_ _ w805 _ _]
          frame "打开连接", Default {
            n560 = Enqueue Element(queue=w794, element=enum16{"打开连接", "发送数据", "读取数据", "数据处理", "关闭连接"}."读取数据" ("枚举"), error in (no error)=w793) -> ()  [unwired: 1 in, 3 out]
            n561 = global read "断电保存全局.vi" "VISA resource name"() -> (w804:refnum<visa-resource-name>)
            n562 = global read "断电保存全局.vi" "数据发送通道"() -> (w801:enum16{"TCP", "VISA"})
            n563 = global read "断电保存全局.vi" "baud rate"() -> (w803:u32)
            n564 = global read "断电保存全局.vi" "PORT"() -> (w802:string)
            n565 = global read "断电保存全局.vi" "IP"() -> (w800:string)
            n566 = call "VISATCP组合选择发送.vi"("IP"=w800, "数据发送通道"=w801, "命令"="open", "PORT"=w802, "VISA resource name"=w804, "baud rate"=w803, "error in (no error)"=w796) -> ("错误输出"=w797:errorcluster)  [unwired: 5 in, 3 out]
            n567 = Unbundle By Name(w797) -> ("status"=w791:bool, "code"=w792:i32)
            n568 = Not(x=w791) -> (.not. x?=→"通信状态":bool)
            n569 = global write "全局 数据发送重叠.vi" "掉线指示灯"(w791) -> ()
          }
          frame "发送数据" {
          }
          frame "读取数据" {
            n570 = Get Queue Status(queue=w826, error in (no error)=w825) -> (queue out=w822:refnum<queue>, error out=w821:errorcluster, # elements in queue=w824:i32)  [unwired: 1 in, 5 out]
            n571 = global read "断电保存全局.vi" "数据发送通道"() -> (w833:enum16{"TCP", "VISA"})
            n572 = Equal To 0?(x=w824) -> (x = 0?=w823:bool)
            n573 = case shown="真" w823 {
              tunnel: w822 -> [_ w858]
              tunnel: w821 -> [_ w857]
              frame False {
              }
              frame True {
                n574 = Enqueue Element(queue=w858, element=enum16{"打开连接", "发送数据", "读取数据", "数据处理", "关闭连接"}."读取数据" ("枚举"), error in (no error)=w857) -> ()  [unwired: 1 in, 3 out]
              }
            }
            n575 = call "VISATCP组合选择发送.vi"("数据发送通道"=w833, "命令"="read", "error in (no error)"=w834) -> ("读取缓冲区"=w819:string, "错误输出"=w831:errorcluster)  [unwired: 9 in, 2 out]
            n576 = call "读取数据处理 (子VI).vi"("data out"=w819) -> ("命令编码CN"=w827:string, "数据"=w815:string, "时间QN"=w807:string)  [unwired: 8 in, 4 out]
            n577 = Empty String/Path?(string/path=w819) -> (empty?=w820:bool)
            n578 = case shown="假" w820 {
              tunnel: w819 -> [w854 _]
              tunnel: w807 -> [w851 _]
              frame False {
                n579 = Search/Split String(string=w851, search string/char (-)="QN=" ("搜索字符串/字符(-)")) -> (match + rest of string=w850:string)  [unwired: 1 in, 2 out]
                n580 = global write "全局1.vi" "数据输出"(w854) -> ()
                n581 = global write "全局1.vi" "读取报文显示"(w854) -> ()
                n582 = String Subset(string=w850, offset (0)=3 ("偏移量(0)")) -> (substring=w849:string)  [unwired: 1 in]
                n583 = global write "全局1.vi" "QN"(w849) -> ()
                n584 = call "数据记录.vi"("写入字段"=w854) -> ("连接的字符串"=w855:string)  [unwired: 10 in]
                n585 = Build Array(w855) -> (w856:string[])
                n586 = call "发送数据记录到文档(子VI).vi"("数组"=w856) -> ()  [unwired: 9 in, 1 out]
              }
              frame True {
              }
            }
            n587 = Search/Split String(string=w827, search string/char (-)="CN=" ("搜索字符串/字符(-)")) -> (match + rest of string=w828:string)  [unwired: 1 in, 2 out]
            n588 = String Subset(string=w828, offset (0)=3 ("偏移量(0)")) -> (substring=w813:string)  [unwired: 1 in]
            n589 = Empty String/Path?(string/path=w813) -> (empty?=w816:bool)
            n590 = Not Equal?(x=w813, y="9013") -> (x != y?=w810:bool)
            n591 = Not Equal?(x=w813, y="9014") -> (x != y?=w809:bool)
            n592 = Not(x=w816) -> (.not. x?=w808:bool)
            n593 = Compound Arithmetic op=AND ("复合运算")(w808, w810, w809) -> (w814:bool)
            n594 = case shown="真" w814 {
              tunnel: w818 -> [_ w848]
              tunnel: w817 -> [_ w847]
              tunnel: w815 -> [_ w846]
              tunnel: w813 -> [_ w837]
              tunnel: w807 -> [_ w842]
              tunnel: w806 -> [_ w841]
              tunnel: w805 -> [_ w840]
              frame False {
              }
              frame True {
                n595 = global write "全局1.vi" "数据"(w846) -> ()
                n596 = Search/Split String(string=w842, search string/char (-)="QN=" ("搜索字符串/字符(-)")) -> (match + rest of string=w845:string)  [unwired: 1 in, 2 out]
                n597 = global write "全局1.vi" "命令编码CN"(w837) -> ()
                n598 = String Subset(string=w845, offset (0)=3 ("偏移量(0)")) -> (substring=w836:string)  [unwired: 1 in]
                n599 = Bundle By Name(cluster=cluster{"命令编码CN":string, "QN":string} {"命令编码CN"="", "QN"=""}, "命令编码CN"=w837, "QN"=w836) -> (w838:cluster{"命令编码CN":string, "QN":string})
                n600 = Enqueue Element At Opposite End(queue=w848, element="反控命令" ("元素"), error in (no error)=w847) -> ()  [unwired: 1 in, 3 out]
                n601 = Enqueue Element(queue=w841, element=w838, error in (no error)=w840) -> ()  [unwired: 1 in, 3 out]
              }
            }
          }
          frame "数据处理" {
          }
          frame "关闭连接" {
            n602 = global read "断电保存全局.vi" "数据发送通道"() -> (w866:enum16{"TCP", "VISA"})
            n603 = Enqueue Element(queue=w861, element=enum16{"打开连接", "发送数据", "读取数据", "数据处理", "关闭连接"}."打开连接" ("枚举"), error in (no error)=w860) -> ()  [unwired: 1 in, 3 out]
            n604 = call "VISATCP组合选择发送.vi"("数据发送通道"=w866, "命令"="close", "error in (no error)"=w864) -> ("错误输出"=w865:errorcluster)  [unwired: 9 in, 3 out]
            n605 = call <vilib>:"Clear Errors.vi"("error in (no error)"=w865) -> ("error out"=w863:errorcluster)  [unwired: 5 in, 1 out]
          }
        }
        n606 = local read "状态信息"() -> (w786:T5)
        n607 = Bundle By Name(cluster=w786, "TCP服务端掉线计数"=0, "1st Error to Convert"=w784, "步骤"=w783) -> (→"状态信息":T5)
      }
      frame Error {
        n608 = Unbundle By Name(w872) -> ("code"=w871:i32)
        n609 = case shown="54, 63" w871 {
          tunnel: w870 -> [w879 w895 w906]
          tunnel: w869 -> [w878 w894 w905]
          tunnel: [w877 w892 w904] -> w868
          frame 0, Default {
            n610 = Flush Queue(queue=w879, error in (no error)=w878) -> (queue out=w881:refnum<queue>, error out=w882:errorcluster)  [unwired: 1 out]
            n611 = local read "状态信息"() -> (w876:T5)
            n612 = Enqueue Element(queue=w881, element=enum16{"打开连接", "发送数据", "读取数据", "数据处理", "关闭连接"}."关闭连接" ("枚举"), error in (no error)=w882) -> (error out=w883:errorcluster)  [unwired: 1 in, 2 out]
            n613 = Unbundle By Name(w876) -> ("TCP服务端掉线计数"=w874:i32)
            n614 = Increment(x=w874) -> (x+1=w875:i32)
            n615 = Bundle By Name(cluster=w876, "TCP服务端掉线计数"=w875) -> (w873:T5)
            n616 = local write "状态信息"(w873) -> ()
            n617 = call <vilib>:"Clear Errors.vi"("error in (no error)"=w883) -> ("error out"=w877:errorcluster)  [unwired: 5 in, 1 out]
          }
          frame 54, 63 {
            n618 = Flush Queue(queue=w895, error in (no error)=w894) -> (queue out=w897:refnum<queue>, error out=w898:errorcluster)  [unwired: 1 out]
            n619 = local read "状态信息"() -> (w887:T5)
            n620 = Unbundle By Name(w887) -> ("TCP服务端掉线计数"=w891:i32, "TCP掉线时间节点"=w884:string)
            n621 = Enqueue Element(queue=w897, element=enum16{"打开连接", "发送数据", "读取数据", "数据处理", "关闭连接"}."关闭连接" ("枚举"), error in (no error)=w898) -> (error out=w893:errorcluster)  [unwired: 1 in, 2 out]
            n622 = Less Or Equal?(x=w891, y=1) -> (x <= y?=w889:bool)
            n623 = Increment(x=w891) -> (x+1=w886:i32)
            n624 = case shown="真" w889 {
              tunnel: [w899 w900] -> w888
              tunnel: w884 -> [w899 _]
              frame False {
              }
              frame True {
                n625 = Get Date/Time In Seconds() -> (seconds since 1Jan1904=w901:timestamp)
                n626 = Format Date/Time String(time format string (%c)="%Y%m%d%H%M%S%3u" ("时间格式字符串(%c)"), seconds (now)=w901) -> (date/time string=w903:string)  [unwired: 1 in]
                n627 = call "格式时间字符串.vi"("字符串"=w903) -> ("连接的字符串"=w900:string)  [unwired: 10 in]
              }
            }
            n628 = call <vilib>:"Clear Errors.vi"("error in (no error)"=w893) -> ("error out"=w892:errorcluster)  [unwired: 5 in, 1 out]
            n629 = Bundle By Name(cluster=w887, "TCP服务端掉线计数"=w886, "TCP掉线时间节点"=w888) -> (w885:T5)
            n630 = local write "状态信息"(w885) -> ()
          }
          frame 56 {
            n631 = Flush Queue(queue=w906, error in (no error)=w905) -> (queue out=w908:refnum<queue>, error out=w909:errorcluster)  [unwired: 1 out]
            n632 = Enqueue Element(queue=w908, element=enum16{"打开连接", "发送数据", "读取数据", "数据处理", "关闭连接"}."读取数据" ("枚举"), error in (no error)=w909) -> (error out=w910:errorcluster)  [unwired: 1 in, 2 out]
            n633 = call <vilib>:"Clear Errors.vi"("error in (no error)"=w910) -> ("error out"=w904:errorcluster)  [unwired: 5 in, 1 out]
          }
        }
      }
    }
  }
  n634 = disable-structure shown="禁用" {
    frame Disabled {
      w911 = string[] ["OPEN", "APP数据传输", "EXIT"]
      # "6."
      # "3."
      # "1."
      n635 = call <vilib>:"Application Directory.vi"() -> ("Application Directory"=w924:path)
      n636 = property class="App"() -> ("App.Name"=w914:string)  [unwired: 2 in, 2 out]
      n637 = Build Path(base path=w924, name or relative path="data\\tubiao.ico" ("名称或相对路径")) -> (appended path=w932:path)
      n638 = Current VI's Path() -> (path=w921:path)
      n639 = Build Array(w932) -> (w927:path[])
      n640 = Open VI Reference(vi path=w921) -> (vi reference=w920:refnum<vi>)  [unwired: 5 in, 1 out]
      n641 = invoke class="VI" method="FP.Open"(reference=w920, "Activate"=TRUE ("激活？"), "State"=T23."Standard" ("状态")) -> (error out=w919:errorcluster)  [unwired: 2 in, 4 out]
      n642 = Build Array("Open", w914, "Exit" ("元素")) -> (w912:string[])
      n643 = call <vilib>:"Constructor.vi"("error in"=w919, "IconFilePathList"=w927) -> ("error out"=w931:errorcluster, "NotifyIcon"=w925:refnum<class "NotifyIcon.lvclass">)  [unwired: 8 in]
      n644 = for {
        shift-right: [w990] -> w943
        shift-left: w931 -> [w991]
        tunnel: w912 -> [w989] mode=indexing
        tunnel: w911 -> [w988] mode=indexing
        shift-right: [w986] -> w942
        shift-left: w925 -> [w987]
        # "2."
        n645 = call <vilib>:"InsertMenuItem.vi"("error in"=w991, "ItemTag"=w988, "ItemName"=w989, "NotifyIcon in"=w987) -> ("error out"=w990:errorcluster, "NotifyIcon out"=w986:refnum<class "NotifyIcon.lvclass">)  [unwired: 6 in]
      }
      n646 = Index Array(array=w911) -> (element=w926:string)  [unwired: 1 in]
      n647 = property class="NotifyIcon"(reference=w942, error in=w943, "Public:Visible"=TRUE ("Visible"), "Public:DefaultMenuItem"=w926, "Public:TipText"="平台数据传输系统" ("TipText")) -> (reference out=w939:refnum<class "NotifyIcon.lvclass">, error out=w930:errorcluster, "Public:SelectedItemEvent"=w929:refnum<user-event>)
      n648 = register-events(error in=w930, w929) -> (reference out=w916:refnum<event-registration>, error out=w917:errorcluster)  [unwired: 1 in]
      n649 = while {
        shift-right: [w947] -> w937
        shift-left: w917 -> [w946]
        shift-right: [w948] -> w934
        shift-left: w939 -> [w949]
        shift-right: [w945] -> w935
        shift-left: w916 -> [w950]
        tunnel: [w944] -> _
        stop <- w944 stop-if-true
        n650 = case shown="无错误" w946 {
          selector: w946 -> [w952 w983]
          tunnel: w950 -> [w957 w978]
          tunnel: w949 -> [w956 w979]
          tunnel: [w955 w979] -> w948
          tunnel: [w954 w981] -> w947
          tunnel: [w953 FALSE ("Discard?")] -> w944
          tunnel: [w951 w978] -> w945
          frame No Error {
            n651 = event shown="[1] 前面板关闭？" {
              selector: w957 -> [_ _]
              dyn-events: [_ _] -> w951
              timeout: _ -> [_ _]
              tunnel: w952 -> [w960 w976]
              tunnel: [w960 w975] -> w954
              tunnel: [w959 FALSE ("Discard?")] -> w953
              tunnel: w956 -> [w958 w977]
              tunnel: [w958 w974] -> w955
              event User Event {
                # "5."
                n652 = event-data() -> ("ItemTag"=w961:string)  [unwired: 1 in]
                n653 = case shown="默认" w961 {
                  tunnel: [FALSE TRUE] -> w959
                  frame Default {
                    n654 = Current VI's Path() -> (path=w963:path)
                    n655 = Open VI Reference(vi path=w963) -> (vi reference=w964:refnum<vi>)  [unwired: 5 in, 1 out]
                    n656 = invoke class="VI" method="FP.Open"(reference=w964, "Activate"=TRUE ("激活？"), "State"=T23."Standard" ("状态")) -> ()  [unwired: 2 in, 5 out]
                  }
                  frame "EXIT" {
                  }
                }
              }
              event Panel Close? {
                # "4."
                n657 = event-data() -> ("VIRef"=w970:refnum<vi>)  [unwired: 1 in, 3 out]
                n658 = invoke class="VI" method="FP.Open"(reference=w970, "State"=T23."Hidden" ("状态")) -> ()  [unwired: 3 in, 5 out]
                n659 = call <vilib>:"ShowBalloonTip.vi"("Balloon Icon"=BalloonIcon."Information", "error in"=w976, "Text"="欢迎使用平台数据传输系统", "NotifyIcon in"=w977) -> ("error out"=w975:errorcluster, "NotifyIcon out"=w974:refnum<class "NotifyIcon.lvclass">)  [unwired: 6 in]
                n660 = event-data("Discard?"=TRUE ("放弃？")) -> ()  [unwired: 1 in, 1 out]
              }
            }
          }
          frame Error {
            n661 = call <vilib>:"Simple Error Handler.vi"("error in (no error)"=w983) -> ("error out"=w982:errorcluster)  [unwired: 4 in, 4 out]
            n662 = call <vilib>:"Clear Errors.vi"("error in (no error)"=w982) -> ("error out"=w981:errorcluster)  [unwired: 5 in, 1 out]
          }
        }
      }
      n663 = property class="App"() -> ("App.Kind"=w918:T25)  [unwired: 2 in, 2 out]
      n664 = Unregister For Events(event registration refnum=w935, error in=w937) -> (error out=w938:errorcluster)
      n665 = call <vilib>:"Destructor.vi"("error in"=w938, "NotifyIcon"=w934) -> ("error out"=w933:errorcluster)  [unwired: 9 in]
      n666 = call <vilib>:"Simple Error Handler.vi"("error in (no error)"=w933) -> ("error out"=→"错误输出":errorcluster)  [unwired: 4 in, 4 out]
      n667 = case shown="\"Run Time System\"" w918 {
        tunnel: w933 -> [_ _ _ _ _ _ _]
        frame "invalid app kind", Default {
        }
        frame "Development System" {
          n668 = Stop(stop? (T)=TRUE ("可见")) -> ()
        }
        frame "Run Time System" {
          n669 = Quit LabVIEW(quit? (T)=TRUE ("退出？(T)")) -> ()
        }
        frame "Student Edition" {
        }
        frame "Embedded LabVIEW" {
        }
        frame "Evaluation" {
        }
        frame "Custom" {
        }
      }
    }
    frame Enabled {
    }
  }
